vi "MoD Main-Optimize - HPLC BH-Amination - ReOpt.vi"() -> ()   [LabVIEW 2015]
uses:
  <vilib>/silver_ctls/ArrayMatrixCluster/Real Matrix NI_Silver.ctl
  <vilib>/ni845x/ni845x.llb/ni845xControl.ctl
  <vilib>/MakerHub/LINX/Public/Peripherals/Analog/Analog Read 1 Chan.vi
  <vilib>/MakerHub/LINX/Public/Peripherals/Analog/Analog Read N Chans.vi
  <vilib>/MakerHub/LINX/Public/Peripherals/Digital/Digital Write 1 Chan.vi
  <vilib>/MakerHub/LINX/Private/Local IO/LinxAnalogRead.vi
  <vilib>/MakerHub/LINX/Public/Utilities/Check Channel.vi
  <vilib>/MakerHub/LINX/Public/Peripherals/Digital/Digital Write N Chans.vi
  <vilib>/MakerHub/LINX/Private/Local IO/LinxDigitalWrite.vi
  <vilib>/addons/control/pid/pid.llb/PID Control Input Filter (DBL).vi
  <vilib>/MakerHub/LINX/Private/Utilties/Generate Error.vi
  <vilib>/addons/control/pid/autopid.llb/PID Online Autotuning (Relay Feedback).vi
  <vilib>/Analysis/Matrix/Numeric/Conversions/Array To Matrix - RA2.vi
  <vilib>/ni845x/ni845x.llb/NI-845x Close Device Reference.vi
  <vilib>/addons/control/pid/NI_PID_autopid.lvlib
  <vilib>/addons/control/pid/NI_PID_pid.lvlib
  <vilib>/Analysis/Matrix/NI_Matrix.lvlib
  <vilib>/MakerHub/LINX/LMH-LINX.lvlib
  <instrlib>/Harvard Apparatus PHD Ultra Series/Harvard Apparatus PHD Ultra Series.lvlib
panel:
  out "running?":bool=TRUE
  out "new_reactor_volume":bool[](array[boolean])
  out "new_reactor_length":bool[](array[boolean])
  out "Phase_Sensor_voltage":dbl
  out "P_tot":dbl
  out "pause for ms":bool=TRUE
  out "stop_xl_write":bool=TRUE
  out "Num_exp_till_pause":i32
  out "Syringe_pump?":bool=TRUE
  out "System Error":bool=TRUE
  out "error out":errorcluster
  out "Pump setpoint(ul/min) 6":dbl format="%#_13g"
  out "Pump setpoint(ul/min) 5":dbl format="%#_13g"
  out "Pump setpoint(ul/min) 4":dbl format="%#_13g"
  out "Pump setpoint(ul/min) 3":dbl format="%#_13g"
  out "Pump setpoint(ul/min) 2":dbl format="%#_13g"
  out "Pump setpoint(ul/min) 1":dbl format="%#_13g"
  out "Volume (ul) 5":dbl format="%#_13g"
  out "Volume (ul) 4":dbl format="%#_13g"
  out "Volume (ul) 3":dbl format="%#_13g"
  out "Volume (ul) 2":dbl format="%#_13g"
  out "Volume (ul) 1":dbl format="%#_13g"
  in  "tau 5":dbl format="%#_13g"
  out "tau 4":dbl format="%#_13g"
  out "tau 3":dbl format="%#_13g"
  out "tau 2":dbl format="%#_13g"
  out "tau 1":dbl format="%#_13g"
  out "Reactor Length":dbl format="%#_13g"
  out "Flowrate Sensor 2":dbl format="%#_13g"
  out "Flowrate Sensor 1":dbl format="%#_13g"
  out "Pressure 2":dbl format="%#_13g"
  out "Pressure 1":dbl format="%#_13g"
  out "Temperature Control 5":bool=TRUE
  out "Temperature Control 4":bool=TRUE
  out "Temperature Control 3":bool=TRUE
  out "Temperature Control 2":bool=TRUE
  out "Temperature Control 1":bool=TRUE
  out "Temperature SP 5":dbl format="%#_g'C"
  out "Temperature SP 4":dbl format="%#_g'C"
  out "Temperature SP 3":dbl format="%#_g'C"
  out "Temperature SP 2":dbl format="%#_g'C"
  out "Temperature SP 1":dbl format="%#_g'C"
  in  "Bay Temperature 5":dbl
  in  "SSR Duration 5":dbl
  in  "SSR Duration 4":dbl
  in  "SSR Duration 3":dbl
  in  "SSR Duration 2":dbl
  in  "SSR Duration 1":dbl
  in  "Total Product Amount":dbl=1.0 format="%#_gml"
  out "Setup Error":bool=TRUE
  out "Error Message":string
  out "ID CTR":i32
  in  "Tab Control":T1(tab)
  out "Reagent pic 5":picture
  in  "reagent name 5":string="toluene"
  out "Reagent Pic 4":picture
  in  "reagent name 4":string="sodium hydroxide"
  out "Reagent Pic 3":picture
  in  "reagent  name 3":string="1470372-59-8"
  in  "Product name":string="101-70-2"
  in  "reagent name 1":string="4-bromoanisole"
  out "Reagent Pic 1":picture
  in  "Vr5":dbl format="%#_guL"
  in  "Vr4":dbl format="%#_guL"
  in  "Vr3":dbl format="%#_guL"
  in  "Vr2":dbl format="%#_guL"
  in  "Vr1":dbl format="%#_guL"
  in  "System decide help Button":bool
  in  "Reaction Scheme Confirm":bool
  in  "Synthesis Route Array":string[][](array[string])=[["4-bromoanisole + naphtalene (0.5M)", "1", "PhB(OH)2", "", "", ""], ["p-anisidine", "1", "-", "-", "-", "-"], ["Brettphos PdG3", "0.0025", "-", "-", "-", "-"], ["NaOH", "1", "-", "-", "-", "-"], ["Toluene", "8", "-", "-", "-", "-"], ["Water", "8", "-", "-", "-", "-"]]
  in  "System decide help Button 2":bool
  out "Setup Confirm":bool=TRUE
  in  "BAY 1":u16(ring) items=["               Bypass", "         Heated Reactor", "    Small Heated Reator", "         Cooled Reactor", "      Packed Bed Reactor", "          Photo Reactor", "             Separator"]
  in  "BAY 5":u16(ring)=6 items=["               Bypass", "         Heated Reactor", "    Small Heated Reactor", "         Cooled Reactor", "     Packed Bed Reactor", "         Photo Reactor", "             Separator"]
  in  "BAY 4":u16(ring) items=["                Bypass", "         Heated Reactor", "    Small Heated Reactor", "         Cooled Reactor", "     Packed Bed Reactor", "         Photo Reactor", "             Separator"]
  in  "BAY 3":u16(ring)=1 items=["               Bypass", "         Heated Reactor", "    Small Heated Reactor", "         Cooled Reactor", "     Packed Bed Reactor", "          Photo Reactor", "             Separator"]
  in  "BAY 2":u16(ring) items=["               Bypass", "         Heated Reactor", "    Small Heated Reactor", "         Cooled Reactor", "      Packed Bed Reactor", "          Photo Reactor", "             Separator"]
  out "Reagent Pic 2":picture
  out "Product Pic":picture
  in  "reagent name 2":string="p-anisidine"
  in  "reagent name 6":string="water"
  out "Reagent Pic 6":picture
  in  "System Parameters Help Button":bool
  out "Setup Confirm 2":bool
  in  "System Parameters Confirm Button":bool
  in  "Bay Parameters":T2={"Bay 1 "={"Pump 1 Flowrate"=0.0, "optimize_temp"=FALSE, "optimize_tau"=TRUE, "Run at set flowrate"=FALSE, "Pump 2 Flowrate"=0.0, "Temperature Params"=[40.0, 100.0, 100.0], "pump params 1"=[16.3, 65.9, 325.0], "pump params 2"=[16.3, 65.9, 325.0], "Temperature"=0.0, "Run at set temperature"=FALSE}, "Bay 2 "={"Pump 3 Flowrate"=0.5, "optimize_temp"=FALSE, "optimize_tau"=FALSE, "Run at set flowrate"=TRUE, "Temperature Params"=[40.0, 100.0, 100.0], "Resisdence time params"=[0.1, 2.0, 650.0], "pump_at_ratio"=FALSE, "pump_num_ratio"=4.0, "Temperature"=0.0, "Run at set temperature"=FALSE}, "Bay 3 "={"Pump 4 Flowrate"=100.0, "optimize_temp"=FALSE, "optimize_tau"=TRUE, "Run at set flowrate"=FALSE, "Temperature Params"=[40.0, 100.0, 100.0], "Resisdence time params"=[16.3, 65.9, 0.0], "pump_at_ratio"=FALSE, "pump_num_ratio"=0.0, "Temperature "=100.0, "Run at set temperature"=TRUE}, "Bay 4 "={"Pump 5 Flowrate"=40.0, "Run at set flowrate"=FALSE, "optimize_temp"=FALSE, "optimize_tau"=FALSE, "Resisdence time params"=[40.6, 406.0, 225.0], "Temperature Params"=[40.0, 100.0, 80.0], "pump_at_ratio"=TRUE, "pump_num_ratio"=1.0, "Temperature"=0.0, "Run at set temperature"=FALSE}, "Bay 5 "={"Pump 6 Flowrate"=0.0, "Run at set flowrate"=FALSE, "optimize_temp"=FALSE, "optimize_tau"=FALSE, "Resisdence time params"=[7.62, 114.27, 0.0], "Temperature Params"=[0.0, 0.0, 0.0], "pump_at_ratio"=TRUE, "pump_num_ratio"=0.5, "Temperature"=0.0, "Run at set temperature"=FALSE}, "Excel File Name"="C:\\Users\\HPLC\\Dropbox (MIT)\\MoD Files\\Data\\BHamination07252017", "hplc File Name"="C:\\Chem32\\1\\Data\\MOD", "Matlab File"="C:\\Users\\HPLC\\Dropbox (MIT)\\MoD Files\\Data\\BHamination07252017", "Syringe for Pump 2?"=TRUE, "Num_conditons_per_wait"=2.0, "Continue from previous optimization?"=FALSE, "Total Number of Experiments 2"=15.0, "Hplc Wait time(min)"=5.0, "increas_decrease_hplc_peak"=TRUE, "Internal Standard?"=TRUE, "ISTD start"=3.7, "ISTD end"=5.0, "hplc_start"=3.0, "hplc_end"=4.0, "throughput_yield"=TRUE} {"Hplc Wait time(min)" format="%#_13g"; "Bay 5"."Temperature Params" format="%#_g'C"; "Bay 4"."Temperature Params" format="%#_g'C"; "Bay 3"."Temperature Params" format="%#_g'C"; "Bay 2"."Temperature Params" format="%#_g'C"; "Bay 1"."Temperature Params" format="%#_g'C"}
  out "System Confirm Not Clicked":string
  out "best_exp_num":dbl=1.0
  out "temperature_best":dbl[](array[numeric])
  out "Flowrates(ul/min)_best":dbl[](array[numeric])
  out "System Status":u16(ring)=2 caption="Sy" items=["System  Error", "System Running", "System Standby"]
  out "Current Experiment":dbl=1.0
  out "Total Number of Experiments":dbl=33.0
  out "Phase Sensor Chart":T3(graph)
  out "HPLC Analysis":bool
  out "Equlibrating Temperature":bool
  out "Flushing System":bool
  out "Calculate condition":bool
  out "Temperature 5":dbl format="%#_g'C"
  out "Temperature 4":dbl format="%#_g'C"
  out "Temperature 3":dbl format="%#_g'C"
  out "Temperature 2":dbl format="%#_g'C"
  out "Temperature 1":dbl format="%#_g'C"
  out "Flowrate Chart":T4(graph)
  out "Teperature Chart":T3(graph)
  out "Pump Setpoints Chart":T3(graph)
  out "Pressure Chart":T3(graph)
  out "Optimization_loop_index":i32
  out "curr_wait_time":dbl
  out "total_flush_time":dbl
  out "Temp SS? 5":bool=TRUE
  out "Temp SS? 4":bool=TRUE
  out "Temp SS? 3":bool=TRUE
  out "Temp SS? 2":bool=TRUE
  out "Temp SS? 1":bool=TRUE
  out "System Flushed?":bool
  out "stop_button clicked":bool
  out "experiment history":T5
  in  "Number of System Flushes per condtion":dbl=2.5
  in  "calculate volume 3":bool
  in  "calculate volume 2":bool=TRUE
  in  "calculate volume 1":bool=TRUE
  in  "calculate volume 4":bool
  in  "calculate volume 5":bool
  in  "Extra system dead volume":dbl format="%#_gul"
  in  "new reactor length? 1":bool
  in  "tube_length(in)":dbl[](array[numeric])=[188.0, 188.0, 10.0, 10.0, 10.0]
  out "Pause Before Analysis":bool
  out "Chiller COMM Port":bool
  out "Arduino COMM Port 2":bool
  out "Temperature Sensor COMM Port":bool
  out "Flow Rate":bool
  out "Pressure":bool
  out "Pump COMM Port":bool
  in  "COMM Port :: Milligat Pumps":refnum<visa-resource-name>="COM10"
  in  "Arduino COMM Port":refnum<visa-resource-name>="COM3"
  in  "Sample Valve COMM::Port":refnum<visa-resource-name>="COM6"
  in  "COMM Port:: Harvard Syringe Pump":refnum<visa-resource-name>="COM5"
  in  "tube_id(in)":enum16{".01", ".02", ".03", ".04"}[](array[ring])=[enum.".03", enum.".03", enum.".03", enum.".03", enum.".03"]
  out "Total System Resisdence Time(min)":dbl
  in  "Debug_run_button":bool
  in  "new reactor length? 2":bool
  in  "new reactor length? 3":bool
  in  "new reactor length? 4":bool
  in  "new reactor length? 5":bool
  in  "IR Sensor Device":T6="USB0::0x3923::0x7514::01B3FF21::RAW"
  out "Stop":bool=TRUE
  in  "Run_Stop_cluster":T7
  # "Molecules on Demand"
  # "Synthetic Route"
  # "5"
  # "6"
  # "4"
  # "Product"
  # "1"
  # "2"
  # "3"
  # "Reagent List"
  # "Concentration(M)"
  # "Molecule"
  # "1"
  # "1"
  # "2"
  # "2"
  # "3"
  # "3"
  # "4"
  # "4"
  # "5"
  # "6"
  # "5"
  # "6"
  # "Product"
  # "Reactor Volume:"
  # "Optimization Parameters"
  # "Pause after"
  # "Experiments"
  # "Optimize for"
  # "to"
  # "of HPLC Peak from"
  # "from"
  # "to"
  # "min"
  # "min"
  # "HPLC runtime"
  # "# Iterations"
  # "Reporting"
  # "Excel Output File Name"
  # "HPLC File Path"
  # "MATLAB File Path"
  # "Temperature"
  # "Flowrate(ul/min)"
  # "Lower Bound"
  # "Upper Bound"
  # "Optimize?"
  # "-or-"
  # "Run at"
  # "times incoming flow"
  # "Setpoint"
  # "Temperature"
  # "Flowrate(ul/min)"
  # "Lower Bound"
  # "Upper Bound"
  # "Optimize?"
  # "-or-"
  # "Run at"
  # "times incoming flow"
  # "Setpoint"
  # "Temperature"
  # "Flowrate(ul/min)"
  # "Lower Bound"
  # "Upper Bound"
  # "Optimize?"
  # "-or-"
  # "Run at"
  # "times incoming flow"
  # "Setpoint"
  # "Temperature"
  # "Flowrate 3 (ul/min)"
  # "Lower Bound"
  # "Upper Bound"
  # "Optimize?"
  # "-or-"
  # "Run at"
  # "times incoming flow"
  # "Setpoint"
  # "Temperature"
  # "Flowrate 1(ul/min)"
  # "Flowrate 2(ul/min)"
  # "Lower Bound"
  # "Upper Bound"
  # "Optimize?"
  # "Setpoint"
  # "Pressure (psi)"
  # "System Status"
  # "Temperature('C)"
  # "BAY"
  # "1"
  # "2"
  # "3"
  # "4"
  # "5"
  # "Pump Flowrate Setpoint(ul/min)"
  # "Flowrate (ul/min)"
  # "Phase Sensor"
  # "Current Experiment"
  # "Temperature('C)"
  # "Flowrate(ul/min)"
  # "Exp"
  # "Current Best Condition"
  # "Time to reach steady state:"
  # "Current Wait Time:"
  # "Experimental Steps"
  # "Calculated New Conditions"
  # "Steady State"
  # "Analyzed HPLC"
  # "Equilibrated Temperature"
  # "Tube Length (cm)"
  # "Bay"
  # "Tube ID (in)"
  # "Calculate Volume"
  # "Use new tube length"
  # "1."
  # "2."
  # "3."
  # "4."
  # "5."
  # "Reactor Lengths\n*Heated Reactor - 188cm * Small Reactor - 99cm * Bypass - 10cm * Separator - *"
  # "All Experimental Data"
  # "P1"
  # "P2"
  # "P3"
  # "P4"
  # "P5"
  # "P6"
  # "T1"
  # "T2"
  # "T3"
  # "T4"
  # "T5"
  # "Obj_fun"
  # "HPLC_Data"
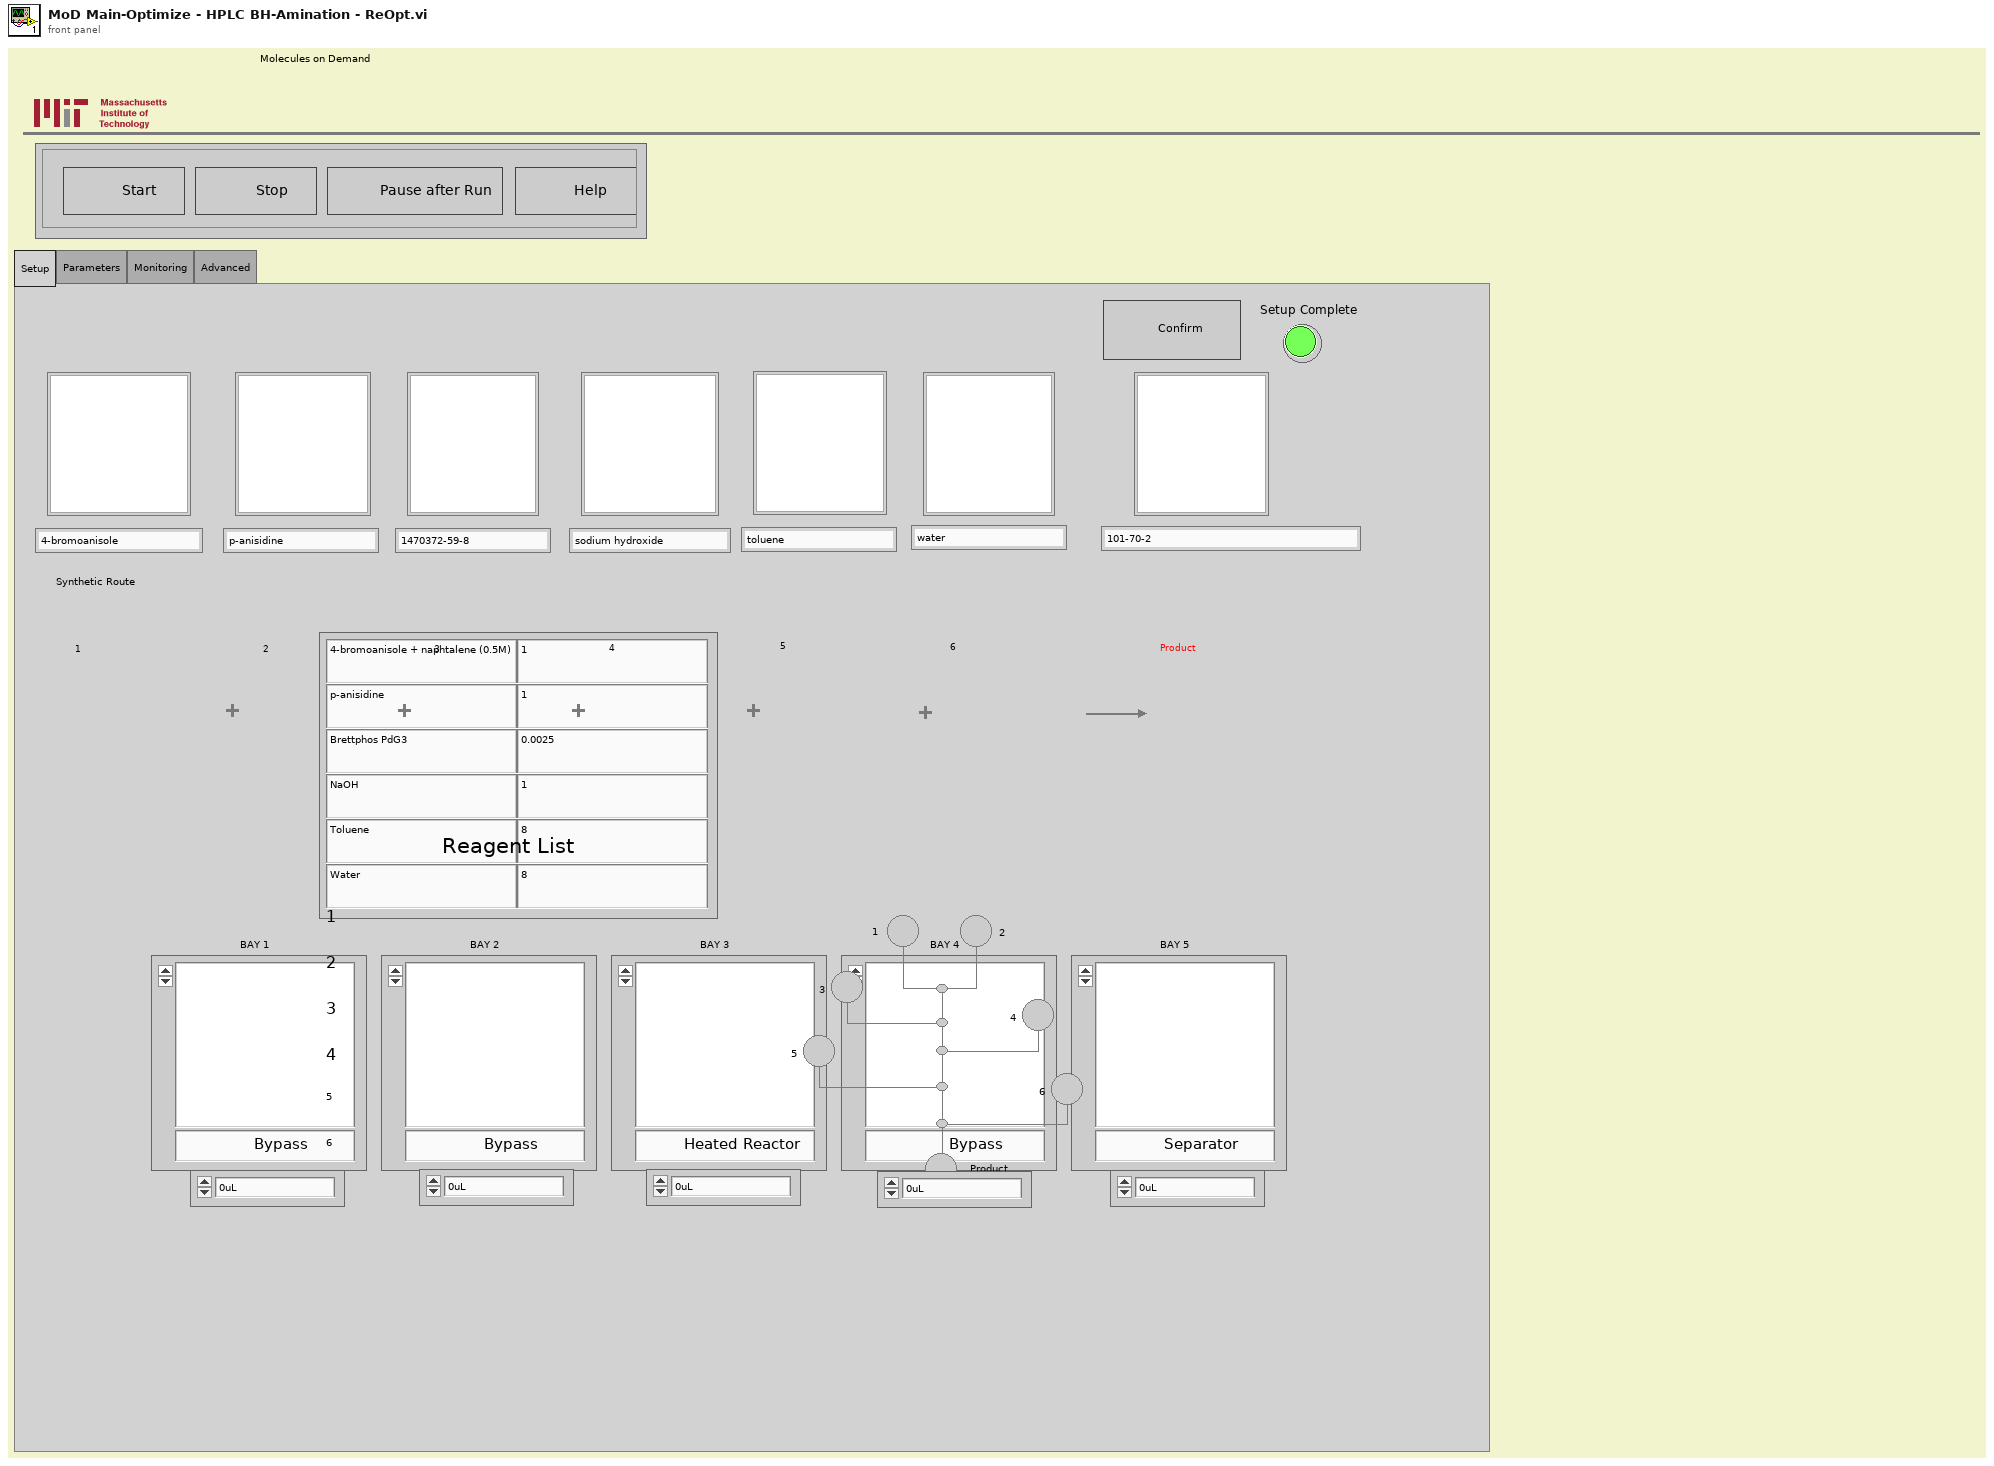
[diagram p1: front panel]
types:
  T1 = enum32{"Setup", "Parameters", "Monitoring", "Advanced"}
  T2 = cluster{"Bay 1 ":cluster{"Pump 1 Flowrate":dbl, "optimize_temp":bool, "optimize_tau":bool, "Run at set flowrate":bool, "Pump 2 Flowrate":dbl, "Temperature Params":dbl[], "pump params 1":dbl[], "pump params 2":dbl[], "Temperature":dbl, "Run at set temperature":bool}, "Bay 2 ":cluster{"Pump 3 Flowrate":dbl, "optimize_temp":bool, "optimize_tau":bool, "Run at set flowrate":bool, "Temperature Params":dbl[], "Resisdence time params":dbl[], "pump_at_ratio":bool, "pump_num_ratio":dbl, "Temperature":dbl, "Run at set temperature":bool}, "Bay 3 ":cluster{"Pump 4 Flowrate":dbl, "optimize_temp":bool, "optimize_tau":bool, "Run at set flowrate":bool, "Temperature Params":dbl[], "Resisdence time params":dbl[], "pump_at_ratio":bool, "pump_num_ratio":dbl, "Temperature ":dbl, "Run at set temperature":bool}, "Bay 4 ":cluster{"Pump 5 Flowrate":dbl, "Run at set flowrate":bool, "optimize_temp":bool, "optimize_tau":bool, "Resisdence time params":dbl[], "Temperature Params":dbl[], "pump_at_ratio":bool, "pump_num_ratio":dbl, "Temperature":dbl, "Run at set temperature":bool}, "Bay 5 ":cluster{"Pump 6 Flowrate":dbl, "Run at set flowrate":bool, "optimize_temp":bool, "optimize_tau":bool, "Resisdence time params":dbl[], "Temperature Params":dbl[], "pump_at_ratio":bool, "pump_num_ratio":dbl, "Temperature":dbl, "Run at set temperature":bool}, "Excel File Name":string, "hplc File Name":string, "Matlab File":string, "Syringe for Pump 2?":bool, "Num_conditons_per_wait":dbl, "Continue from previous optimization?":bool, "Total Number of Experiments 2":dbl, "Hplc Wait time(min)":dbl, "increas_decrease_hplc_peak":bool, "Internal Standard?":bool, "ISTD start":dbl, "ISTD end":dbl, "hplc_start":dbl, "hplc_end":dbl, "throughput_yield":bool}
  T3 = cluster{"[0]":dbl, "[1]":dbl, "[2]":dbl, "[3]":dbl, "[4]":dbl, "[5]":dbl, "[6]":dbl, "[7]":dbl, "[8]":dbl}
  T4 = cluster{"[0]":i32, "[1]":i32, "[2]":i32, "[3]":i32, "[4]":i32, "[5]":i32, "[6]":i32, "[7]":i32, "[8]":i32}
  T5 = typedef "Real Matrix NI_Silver.ctl" = dbl[][]
  T6 = typedef "ni845xControl.ctl" = refnum<k21>
  T7 = cluster{"Stop":bool, "Run":bool, "Stop Run Button":bool, "Help Button":bool}
  T8 = cluster{"Proportional gain Kc":dbl, "Integral time Ti (sec)":dbl, "Derivative time Ti (sec)":dbl}
  T9 = cluster{"type of controller":enum16{"P", "PI", "PID"}, "relay cycles":i32, "relay amplitude":dbl, "control specifications":enum16{"Fast", "Normal", "Slow"}, "PV noise level":dbl}
  T10 = typedef "LMH-LINX.lvlib/LINX Ref.ctl" = cluster{"IO":T11, "Interface":T12, "LINX Device Config":T13}
  T11 = typedef "LMH-LINX.lvlib/Platform.ctl" = enum16{"Remote", "Local"}
  T12 = typedef "LMH-LINX.lvlib/Interface.ctl" = enum16{"Serial", "TCP"}
  T13 = typedef "LMH-LINX.lvlib/Device.lvlib/LINX Device Config.ctl" = cluster{"Interface":T12, "COM Port":refnum<visa-resource-name>, "TCP Configuration":T14, "Device Family":u8, "Device ID":u8, "Device Name":string, "TCP Ref":refnum<k5>, "Channels":T15}
  T14 = typedef "LMH-LINX.lvlib/Device.lvlib/TCP Config.ctl" = cluster{"IP Address":string, "Port":u16}
  T15 = typedef "LMH-LINX.lvlib/Channels.ctl" = cluster{"DI":u8[], "DO":u8[], "AI":u8[], "AO":u8[], "PWM":u8[], "QE":u8[], "UART":u8[], "I2C 2":u8[], "SPI":u8[], "CAN":u8[], "Servo":u8[], "AI Ref (V)":dbl, "AI Resolution (Bits)":u8, "AO Ref (V)":dbl, "AO Resolution (Bits)":u8}
  T16 = typedef "imagedata.ctl" = cluster{"image type":i32, "image depth":i32, "image":u8[], "mask":u8[], "colors":u32[], "Rectangle":cluster{"left":i16, "top":i16, "right":i16, "bottom":i16}}
  T17 = cluster{"proportional gain (Kc)":dbl, "integral time (Ti, min)":dbl, "derivative time (Td, min)":dbl}
  T18 = typedef "NI_Matrix.lvlib/RealMatrix.ctl" = dbl[][]
  T19 = enum16{"Left Button", "Center Button", "Right Button", "Window Close"}
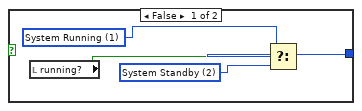
[diagram p3: hidden frame]
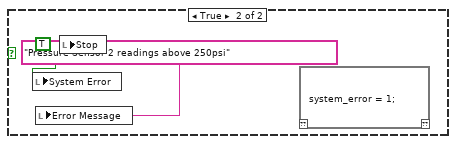
[diagram p4: hidden frame]
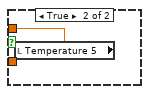
[diagram p6: hidden frame]
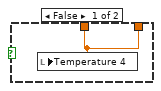
[diagram p7: hidden frame]
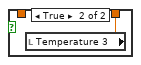
[diagram p8: hidden frame]
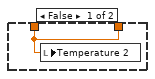
[diagram p9: hidden frame]
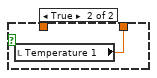
[diagram p10: hidden frame]
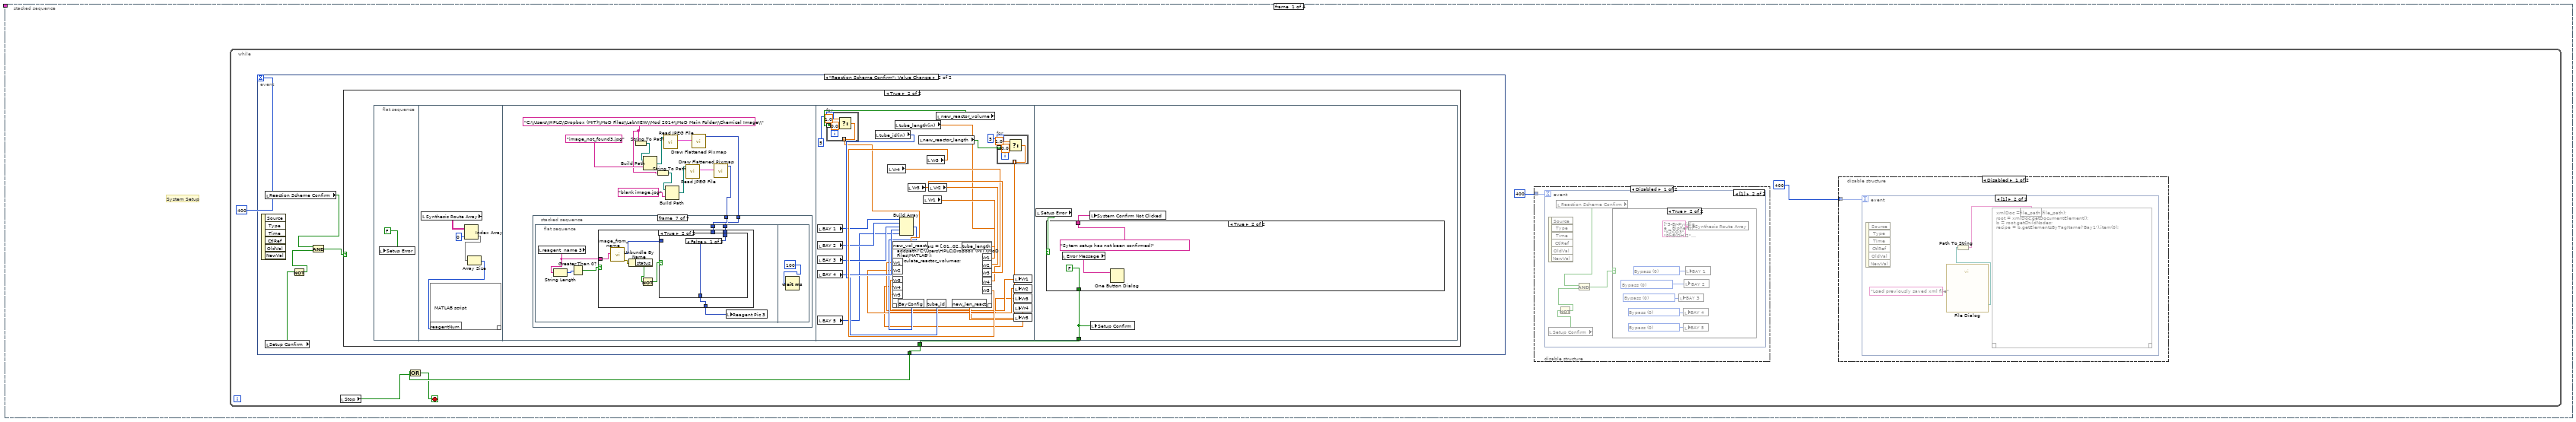
[diagram p11: hidden frame]
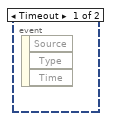
[diagram p12: hidden frame]
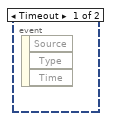
[diagram p14: hidden frame]
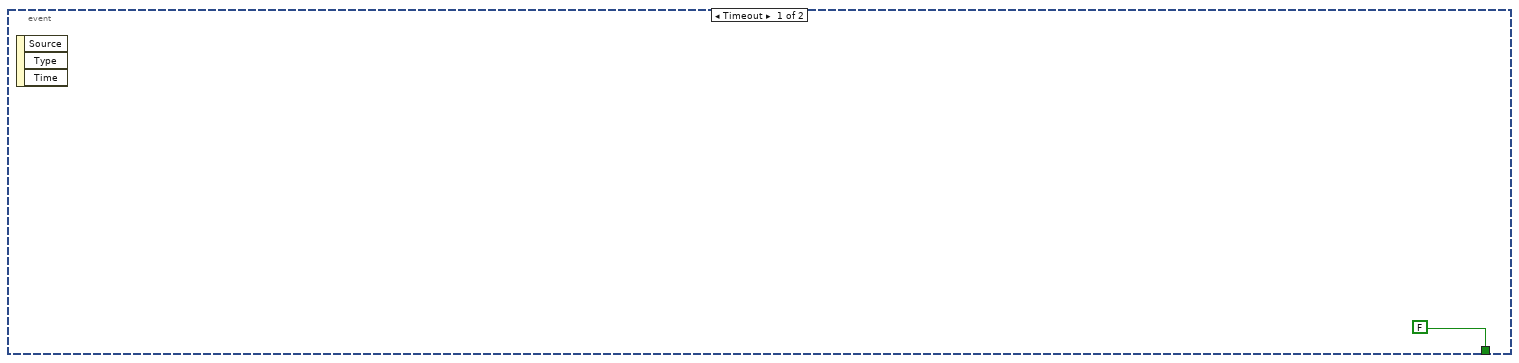
[diagram p17: hidden frame]
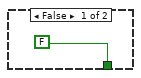
[diagram p18: hidden frame]
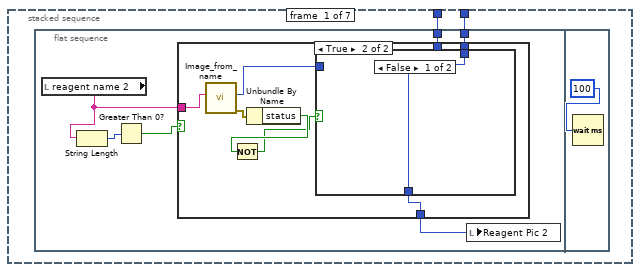
[diagram p19: hidden frame]
diagram:
  # "Assume User always uses the first bay first"
  n1 = flat-sequence {
    tunnel: ["COMM Port :: Milligat Pumps"] -> w9
    tunnel: ["Arduino COMM Port"] -> w8
    tunnel: [w11] -> w5
    tunnel: ["Bay Parameters"] -> w4
    tunnel: [w60] -> w10
    tunnel: w9 -> [w60]
    tunnel: w8 -> [w48]
    tunnel: [w54] -> w7
    tunnel: [w52] -> w6
    tunnel: w5 -> [w52]
    tunnel: w4 -> [w50]
    tunnel: [w47] -> w3
    tunnel: w10 -> [w66]
    tunnel: w7 -> [w65]
    tunnel: w6 -> [w63]
    tunnel: w3 -> [w61]
    tunnel: [w61] -> w1
    tunnel: [w1358] -> w2
    tunnel: w1 -> [w1358]
    tunnel: w2 -> [w1359]
    frame #0 {
      w36 = FALSE ("Equlibrating Temperature")
      n2 = script code="TempArr1=[23 23 23 23 23 23 23 23 23 23]';\nTempArr2=[23 23 23 23 23 23 23 23 23 23]';\nTempArr3=[23 23 23 23 23 23 23 23 23 23]';\nTempArr4=[23 23 23 23 23 23 23 23 23 23]';\nTempArr5=[23 23 23 23 23 23 23 23 23 23]';\ntemp_error1 =0;\ntemp_error2 =0;\ntemp_error3 =0;\ntemp_error4 =0;\ntemp_error5 =0;\ntemp_check1 = 0;\ntemp_check2 = 0;\ntemp_check3 = 0;\ntemp_check4 = 0;\ntemp_check5 = 0;\nT1=23;\nT2=23;\nT3=23;\nT4=23;\nT5=23;"() -> ()  [unwired: 1 in, 1 out]
      n3 = Build Array("calculate volume 1", "calculate volume 2", "calculate volume 3", "calculate volume 4", "calculate volume 5") -> (→"new_reactor_volume":bool[])
      n4 = Build Array("new reactor length? 1", "new reactor length? 2", "new reactor length? 3", "new reactor length? 4", "new reactor length? 5") -> (→"new_reactor_length":bool[])
      n5 = call <vilib>:"Initialize.vi"("VISA resource name"="COMM Port:: Harvard Syringe Pump") -> ("VISA resource name out"=w11:refnum<visa-resource-name>)  [unwired: 9 in, 1 out]
      "Stop" <- FALSE ("Stop")
      "ID CTR" <- 0
      "Setup Confirm" <- FALSE ("Setup Confirm")
      "Error Message" <- "System shutdown sucessfully. No errors to report." ("Error Message")
      "Setup Error" <- FALSE ("Setup Error")
      "Reactor Length" <- 10.5
      "System Error" <- FALSE ("System Error")
      "Num_exp_till_pause" <- 0 ("Num_exp_till_pause")
      "Equlibrating Temperature" <- w36
      "Calculate condition" <- w36
      "Flushing System" <- w36
      "HPLC Analysis" <- w36
      "stop_xl_write" <- FALSE ("stop_xl_write")
      "Pump setpoint(ul/min) 1" <- 0.0 ("Pump setpoint(ul/min) 1")
      "Pump setpoint(ul/min) 2" <- 0.0 ("Pump setpoint(ul/min) 2")
      "Pump setpoint(ul/min) 4" <- 0.0 ("Pump setpoint(ul/min) 4")
      "Pump setpoint(ul/min) 6" <- 0.0 ("Pump setpoint(ul/min) 6")
      "Pump setpoint(ul/min) 3" <- 0.0 ("Pump setpoint(ul/min) 3")
      "Pump setpoint(ul/min) 5" <- 0.0 ("Pump setpoint(ul/min) 5")
      "pause for ms" <- FALSE ("pause for ms")
      "Setup Confirm 2" <- FALSE ("Setup Confirm 2")
      "running?" <- FALSE ("running?")
    }
    frame #1 {
      w49 = FALSE
      w59 = 23
      (unwired) path "C:/Users/User1/Documents/Lab/MoD/Images"
      n6 = disable-structure shown="Disabled" {
        frame Disabled {
          n7 = local read "BAY 2"() -> ()  [unwired: 1 out]
          n8 = local read "BAY 3"() -> ()  [unwired: 1 out]
          n9 = local read "BAY 4"() -> ()  [unwired: 1 out]
          n10 = local read "BAY 5"() -> ()  [unwired: 1 out]
          n11 = local read "BAY 1"() -> ()  [unwired: 1 out]
        }
        frame Enabled {
        }
      }
      n12 = local write "Debug_run_button"(TRUE) -> ()
      n13 = call <vilib>:"Initialize.vi"("Serial Port"=w48) -> ("LINX Resource"=w47:T10)  [unwired: 8 in, 2 out]
      n14 = local write "System Parameters Confirm Button"(w49) -> ()
      n15 = local write "Setup Confirm 2"(w49) -> ()
      n16 = Unbundle By Name(w50) -> ("Syringe for Pump 2?"=→"Syringe_pump?":bool)
      n17 = local write "Temperature 1"(w59) -> ()
      n18 = local write "Temperature 2"(w59) -> ()
      n19 = local write "Temperature 3"(w59) -> ()
      n20 = local write "Temperature 4"(w59) -> ()
      n21 = local write "Temperature 5"(w59) -> ()
      n22 = local write "Temperature SP 1"(w59) -> ()
      n23 = local write "Temperature SP 2"(w59) -> ()
      n24 = local write "Temperature SP 3"(w59) -> ()
      n25 = local write "Temperature SP 4"(w59) -> ()
      n26 = local write "Temperature SP 5"(w59) -> ()
      n27 = Current VI's Path() -> (path=w58:path)
      n28 = Strip Path(path=w58) -> (stripped path=w56:path)  [unwired: 1 out]
      n29 = Strip Path(path=w56) -> (stripped path=w55:path)  [unwired: 1 out]
      n30 = Build Path(base path=w55, name or relative path="MATLAB") -> (appended path=w54:path)
    }
    frame #2 {
      # "Main Help Dialog Popup"
      n31 = while {
        stop <- w1352 stop-if-true
        n32 = event shown="[6] \"Run_Stop_cluster.Run\": Value Change" {
          selector: _ -> [_ _ _ _ _ _ _]
          dyn-events: _ -> [_ _ _ _ _ _ _]
          timeout: 100 -> [_ _ _ _ _ _ _]
          event Timeout {
            n33 = event-data() -> ()  [unwired: 1 in, 3 out]
          }
          event "Run_Stop_cluster.Help Button": Value Change {
            n34 = local read "Run_Stop_cluster"() -> (w1355:T7)
            n35 = event-data() -> ()  [unwired: 1 in, 4 out]
            n36 = Unbundle By Name(w1355) -> ("Help Button"=w1354:bool)
            n37 = case shown="True" w1354 {
              frame False {
              }
              frame True {
                n38 = call "help.vi"() -> ()  [unwired: 11 in]
              }
            }
          }
          event "System decide help Button": Value Change {
            n39 = event-data() -> ()  [unwired: 1 in, 5 out]
            n40 = call "help_synthesis_man-auto_instructions.vi"() -> ()  [unwired: 12 in]
          }
          event "System Parameters Help Button": Value Change {
            n41 = event-data() -> ()  [unwired: 1 in, 5 out]
            n42 = call "help_parameters_setup.vi"() -> ()  [unwired: 12 in]
          }
          event "System decide help Button 2": Value Change {
            n43 = event-data() -> ()  [unwired: 1 in, 5 out]
            n44 = call "help_synthesis_route_instructions.vi"() -> ()  [unwired: 12 in]
          }
          event "Run_Stop_cluster.Stop": Value Change {
            n45 = event-data() -> ()  [unwired: 1 in, 5 out]
            n46 = local write "Stop"(TRUE) -> ()
          }
          event "Run_Stop_cluster.Run": Value Change {
            n47 = event-data() -> ()  [unwired: 1 in, 5 out]
            n48 = local write "running?"(TRUE) -> ()
          }
        }
        n49 = local read "Stop"() -> (w1352:bool)
      }
      n50 = stacked-sequence {
        tunnel: w66 -> [_ _ _ _]
        tunnel: w65 -> [_ w425 _ _]
        tunnel: w63 -> [_ _ _ w592]
        tunnel: w61 -> [_ _ _ w590]
        frame #0 {
          # "System Setup"
          n51 = while {
            stop <- w200 stop-if-true
            n52 = event shown="[1] \"Reaction Scheme Confirm\": Value Change" {
              selector: _ -> [_ _]
              dyn-events: _ -> [_ _]
              timeout: 400 -> [_ _]
              tunnel: [FALSE w220] -> w202
              event Timeout {
                n53 = event-data() -> ()  [unwired: 1 in, 3 out]
              }
              event "Reaction Scheme Confirm": Value Change {
                n54 = event-data() -> ()  [unwired: 1 in, 6 out]
                n55 = local read "Reaction Scheme Confirm"() -> (w224:bool)
                n56 = local read "Setup Confirm"() -> (w222:bool)
                n57 = Not(x=w222) -> (.not. x?=w221:bool)
                n58 = And(x=w224, y=w221) -> (x .and. y?=w223:bool)
                n59 = case shown="True" w223 {
                  tunnel: [FALSE w226] -> w220
                  frame False {
                  }
                  frame True {
                    n60 = flat-sequence {
                      tunnel: [w415] -> w226
                      frame #0 {
                        n61 = local write "Setup Error"(FALSE) -> ()
                      }
                      frame #1 {
                        n62 = local read "Synthesis Route Array"() -> (w230:string[][])
                        n63 = Index Array(array=w230, index (col)=0 ("disabled index (col)")) -> (element=w228:string[])  [unwired: 1 in]
                        n64 = Array Size(array=w228) -> (size(s)=w231:i32)
                        n65 = script code="MATLAB script"("reagentNum"=w231) -> ()  [unwired: 1 in, 1 out]
                      }
                      frame #2 {
                        w234 = "C:\\Users\\HPLC\\Dropbox (MIT)\\MoD Files\\LabVIEW\\Mod 2014\\MoD Main Folder\\Chemical Image\\" ("string")
                        n66 = String To Path(string=w234) -> (path=w240:path)
                        n67 = Build Path(base path=w240, name or relative path="image_not_found3.jpg") -> (appended path=w239:path)
                        n68 = String To Path(string=w234) -> (path=w237:path)
                        n69 = call <vilib>:"Read JPEG File.vi"("path to JPEG file"=w239) -> ("image data"=w242:T16)  [unwired: 1 in, 9 out]
                        n70 = Build Path(base path=w237, name or relative path="blank image.jpg") -> (appended path=w235:path)
                        n71 = call <vilib>:"Read JPEG File.vi"("path to JPEG file"=w235) -> ("image data"=w238:T16)  [unwired: 1 in, 9 out]
                        n72 = call <vilib>:"Draw Flattened Pixmap.vi"("image data"=w242) -> ("new picture"=w233:picture)  [unwired: 3 in, 5 out]
                        n73 = call <vilib>:"Draw Flattened Pixmap.vi"("image data"=w238) -> ("new picture"=w232:picture)  [unwired: 3 in, 5 out]
                        n74 = stacked-sequence {
                          tunnel: w233 -> [w244 w264 w284 w304 w324 w343 w363]
                          tunnel: w232 -> [w243 w263 w283 w303 w323 w344 w364]
                          frame #0 {
                            n75 = flat-sequence {
                              tunnel: w244 -> [w250]
                              tunnel: w243 -> [w248]
                              frame #0 {
                                n76 = local read "reagent name 2"() -> (w246:string)
                                n77 = String Length(string=w246) -> (length=w249:i32)
                                n78 = Greater Than 0?(x=w249) -> (x > 0?=w247:bool)
                                n79 = case shown="True" w247 {
                                tunnel: w250 -> [_ w256]
                                tunnel: w248 -> [w251 _]
                                tunnel: [w251 w255] -> w245
                                tunnel: w246 -> [_ w254]
                                frame False {
                                }
                                frame True {
                                n80 = call "Image_from_name.vi"("Chemical Name"=w254) -> ("error out"=w257:errorcluster, "Downloaded Picture"=w258:picture)  [unwired: 8 in, 1 out]
                                n81 = Unbundle By Name(w257) -> ("status"=w253:bool)
                                n82 = Not(x=w253) -> (.not. x?=w252:bool)
                                n83 = case shown="False" w252 {
                                tunnel: w258 -> [_ w261]
                                tunnel: [w259 w260] -> w255
                                tunnel: w256 -> [w259 _]
                                frame False {
                                }
                                frame True {
                                n84 = call <vilib>:"Draw Flattened Pixmap.vi"("picture"=w261) -> ("new picture"=w260:picture)  [unwired: 8 in]
                                }
                                }
                                }
                                }
                                n85 = local write "Reagent Pic 2"(w245) -> ()
                              }
                              frame #1 {
                                n86 = Wait (ms)(milliseconds to wait=100) -> ()  [unwired: 1 out]
                              }
                            }
                          }
                          frame #1 {
                            n87 = flat-sequence {
                              tunnel: w264 -> [w270]
                              tunnel: w263 -> [w268]
                              frame #0 {
                                n88 = local read "reagent name 1"() -> (w265:string)
                                n89 = String Length(string=w265) -> (length=w269:i32)
                                n90 = Greater Than 0?(x=w269) -> (x > 0?=w267:bool)
                                n91 = case shown="True" w267 {
                                tunnel: w270 -> [_ w276]
                                tunnel: w268 -> [w271 _]
                                tunnel: [w271 w275] -> w266
                                tunnel: w265 -> [_ w274]
                                frame False {
                                }
                                frame True {
                                n92 = call "Image_from_name.vi"("Chemical Name"=w274) -> ("error out"=w277:errorcluster, "Downloaded Picture"=w278:picture)  [unwired: 8 in, 1 out]
                                n93 = Unbundle By Name(w277) -> ("status"=w273:bool)
                                n94 = Not(x=w273) -> (.not. x?=w272:bool)
                                n95 = case shown="True" w272 {
                                tunnel: w278 -> [_ w281]
                                tunnel: [w279 w280] -> w275
                                tunnel: w276 -> [w279 _]
                                frame False {
                                }
                                frame True {
                                n96 = call <vilib>:"Draw Flattened Pixmap.vi"("picture"=w281) -> ("new picture"=w280:picture)  [unwired: 8 in]
                                }
                                }
                                }
                                }
                                n97 = local write "Reagent Pic 1"(w266) -> ()
                              }
                              frame #1 {
                                n98 = Wait (ms)(milliseconds to wait=100) -> ()  [unwired: 1 out]
                              }
                            }
                          }
                          frame #2 {
                            n99 = flat-sequence {
                              tunnel: w284 -> [w290]
                              tunnel: w283 -> [w288]
                              frame #0 {
                                n100 = local read "Product name"() -> (w285:string)
                                n101 = String Length(string=w285) -> (length=w289:i32)
                                n102 = Greater Than 0?(x=w289) -> (x > 0?=w287:bool)
                                n103 = case shown="True" w287 {
                                tunnel: w290 -> [_ w296]
                                tunnel: w288 -> [w291 _]
                                tunnel: [w291 w295] -> w286
                                tunnel: w285 -> [_ w294]
                                frame False {
                                }
                                frame True {
                                n104 = call "Image_from_name.vi"("Chemical Name"=w294) -> ("error out"=w297:errorcluster, "Downloaded Picture"=w298:picture)  [unwired: 8 in, 1 out]
                                n105 = Unbundle By Name(w297) -> ("status"=w292:bool)
                                n106 = Not(x=w292) -> (.not. x?=w293:bool)
                                n107 = case shown="False" w293 {
                                tunnel: w298 -> [_ w301]
                                tunnel: [w299 w300] -> w295
                                tunnel: w296 -> [w299 _]
                                frame False {
                                }
                                frame True {
                                n108 = call <vilib>:"Draw Flattened Pixmap.vi"("picture"=w301) -> ("new picture"=w300:picture)  [unwired: 8 in]
                                }
                                }
                                }
                                }
                                n109 = local write "Product Pic"(w286) -> ()
                              }
                              frame #1 {
                                n110 = Wait (ms)(milliseconds to wait=100) -> ()  [unwired: 1 out]
                              }
                            }
                          }
                          frame #3 {
                            n111 = flat-sequence {
                              tunnel: w304 -> [w310]
                              tunnel: w303 -> [w308]
                              frame #0 {
                                n112 = local read "reagent name 6"() -> (w305:string)
                                n113 = String Length(string=w305) -> (length=w309:i32)
                                n114 = Greater Than 0?(x=w309) -> (x > 0?=w307:bool)
                                n115 = case shown="True" w307 {
                                tunnel: w310 -> [_ w316]
                                tunnel: w308 -> [w311 _]
                                tunnel: [w311 w315] -> w306
                                tunnel: w305 -> [_ w314]
                                frame False {
                                }
                                frame True {
                                n116 = call "Image_from_name.vi"("Chemical Name"=w314) -> ("error out"=w317:errorcluster, "Downloaded Picture"=w318:picture)  [unwired: 8 in, 1 out]
                                n117 = Unbundle By Name(w317) -> ("status"=w312:bool)
                                n118 = Not(x=w312) -> (.not. x?=w313:bool)
                                n119 = case shown="False" w313 {
                                tunnel: w318 -> [_ w321]
                                tunnel: [w319 w320] -> w315
                                tunnel: w316 -> [w319 _]
                                frame False {
                                }
                                frame True {
                                n120 = call <vilib>:"Draw Flattened Pixmap.vi"("picture"=w321) -> ("new picture"=w320:picture)  [unwired: 8 in]
                                }
                                }
                                }
                                }
                                n121 = local write "Reagent Pic 6"(w306) -> ()
                              }
                              frame #1 {
                                n122 = Wait (ms)(milliseconds to wait=100) -> ()  [unwired: 1 out]
                              }
                            }
                          }
                          frame #4 {
                            n123 = flat-sequence {
                              tunnel: w324 -> [w330]
                              tunnel: w323 -> [w328]
                              frame #0 {
                                n124 = local read "reagent name 5"() -> (w325:string)
                                n125 = String Length(string=w325) -> (length=w329:i32)
                                n126 = Greater Than 0?(x=w329) -> (x > 0?=w327:bool)
                                n127 = case shown="True" w327 {
                                tunnel: w330 -> [_ w336]
                                tunnel: w328 -> [w331 _]
                                tunnel: [w331 w335] -> w326
                                tunnel: w325 -> [_ w334]
                                frame False {
                                }
                                frame True {
                                n128 = call "Image_from_name.vi"("Chemical Name"=w334) -> ("error out"=w337:errorcluster, "Downloaded Picture"=w338:picture)  [unwired: 8 in, 1 out]
                                n129 = Unbundle By Name(w337) -> ("status"=w332:bool)
                                n130 = Not(x=w332) -> (.not. x?=w333:bool)
                                n131 = case shown="False" w333 {
                                tunnel: w338 -> [_ w341]
                                tunnel: [w339 w340] -> w335
                                tunnel: w336 -> [w339 _]
                                frame False {
                                }
                                frame True {
                                n132 = call <vilib>:"Draw Flattened Pixmap.vi"("picture"=w341) -> ("new picture"=w340:picture)  [unwired: 8 in]
                                }
                                }
                                }
                                }
                                n133 = local write "Reagent pic 5"(w326) -> ()
                              }
                              frame #1 {
                                n134 = Wait (ms)(milliseconds to wait=100) -> ()  [unwired: 1 out]
                              }
                            }
                          }
                          frame #5 {
                            n135 = flat-sequence {
                              tunnel: w344 -> [w348]
                              tunnel: w343 -> [w347]
                              frame #0 {
                                n136 = local read "reagent name 4"() -> (w345:string)
                                n137 = String Length(string=w345) -> (length=w350:i32)
                                n138 = Greater Than 0?(x=w350) -> (x > 0?=w349:bool)
                                n139 = case shown="True" w349 {
                                tunnel: w347 -> [_ w356]
                                tunnel: w348 -> [w351 _]
                                tunnel: [w351 w355] -> w346
                                tunnel: w345 -> [_ w354]
                                frame False {
                                }
                                frame True {
                                n140 = call "Image_from_name.vi"("Chemical Name"=w354) -> ("error out"=w357:errorcluster, "Downloaded Picture"=w358:picture)  [unwired: 8 in, 1 out]
                                n141 = Unbundle By Name(w357) -> ("status"=w352:bool)
                                n142 = Not(x=w352) -> (.not. x?=w353:bool)
                                n143 = case shown="False" w353 {
                                tunnel: w358 -> [_ w361]
                                tunnel: [w359 w360] -> w355
                                tunnel: w356 -> [w359 _]
                                frame False {
                                }
                                frame True {
                                n144 = call <vilib>:"Draw Flattened Pixmap.vi"("picture"=w361) -> ("new picture"=w360:picture)  [unwired: 8 in]
                                }
                                }
                                }
                                }
                                n145 = local write "Reagent Pic 4"(w346) -> ()
                              }
                              frame #1 {
                                n146 = Wait (ms)(milliseconds to wait=100) -> ()  [unwired: 1 out]
                              }
                            }
                          }
                          frame #6 {
                            n147 = flat-sequence {
                              tunnel: w364 -> [w368]
                              tunnel: w363 -> [w367]
                              frame #0 {
                                n148 = local read "reagent  name 3"() -> (w365:string)
                                n149 = String Length(string=w365) -> (length=w370:i32)
                                n150 = Greater Than 0?(x=w370) -> (x > 0?=w369:bool)
                                n151 = case shown="True" w369 {
                                tunnel: w367 -> [_ w376]
                                tunnel: w368 -> [w371 _]
                                tunnel: [w371 w375] -> w366
                                tunnel: w365 -> [_ w374]
                                frame False {
                                }
                                frame True {
                                n152 = call "Image_from_name.vi"("Chemical Name"=w374) -> ("error out"=w377:errorcluster, "Downloaded Picture"=w378:picture)  [unwired: 8 in, 1 out]
                                n153 = Unbundle By Name(w377) -> ("status"=w372:bool)
                                n154 = Not(x=w372) -> (.not. x?=w373:bool)
                                n155 = case shown="False" w373 {
                                tunnel: w378 -> [_ w381]
                                tunnel: [w379 w380] -> w375
                                tunnel: w376 -> [w379 _]
                                frame False {
                                }
                                frame True {
                                n156 = call <vilib>:"Draw Flattened Pixmap.vi"("picture"=w381) -> ("new picture"=w380:picture)  [unwired: 8 in]
                                }
                                }
                                }
                                }
                                n157 = local write "Reagent Pic 3"(w366) -> ()
                              }
                              frame #1 {
                                n158 = Wait (ms)(milliseconds to wait=100) -> ()  [unwired: 1 out]
                              }
                            }
                          }
                        }
                      }
                      frame #3 {
                        n159 = local read "BAY 1"() -> (w393:u16)
                        n160 = local read "BAY 2"() -> (w392:u16)
                        n161 = local read "BAY 3"() -> (w391:u16)
                        n162 = local read "BAY 4"() -> (w390:u16)
                        n163 = local read "BAY 5"() -> (w389:u16)
                        n164 = local read "tube_id(in)"() -> (w400:enum16{".01", ".02", ".03", ".04"}[])
                        n165 = local read "Vr4"() -> (w403:dbl)
                        n166 = local read "tube_length(in)"() -> (w401:dbl[])
                        n167 = Build Array(w393, w392, w391, w390, w389) -> (w388:u16[])
                        n168 = local read "Vr3"() -> (w404:dbl)
                        n169 = local read "new_reactor_length"() -> (w398:bool[])
                        n170 = local read "Vr1"() -> (w406:dbl)
                        n171 = local read "Vr5"() -> (w402:dbl)
                        n172 = local read "Vr2"() -> (w405:dbl)
                        n173 = local read "new_reactor_volume"() -> (w396:bool[])
                        n174 = for {
                          N: 5 -> [_]
                          tunnel: w396 -> [w410] mode=indexing
                          tunnel: [w407] -> w394 mode=indexing
                          n175 = Select(t=1.0, s=w410, f=0.0) -> (s? t:f=w407:dbl)
                        }
                        n176 = for {
                          N: 5 -> [_]
                          tunnel: w398 -> [w414] mode=indexing
                          tunnel: [w411] -> w397 mode=indexing
                          n177 = Select(t=1.0, s=w414, f=0.0) -> (s? t:f=w411:dbl)
                        }
                        n178 = script code="tube_diameters = [.01,.02,.03,.04];\naddpath('C:\\Users\\HPLC\\Dropbox (MIT)\\MoD Files\\MATLAB');\ncalculate_reactor_volumes;"("BayConfig"=w388, "Vr1"=w406, "Vr2"=w405, "Vr3"=w404, "Vr4"=w403, "Vr5"=w402, "tube_length"=w401, "tube_id"=w400, "new_len_react"=w397, "new_vol_react"=w394) -> ("Vr1"=w387:dbl, "Vr2"=w386:dbl, "Vr3"=w385:dbl, "Vr4"=w384:dbl, "Vr5"=w383:dbl)  [unwired: 1 in, 1 out]
                        n179 = local write "Vr1"(w387) -> ()
                        n180 = local write "Vr2"(w386) -> ()
                        n181 = local write "Vr3"(w385) -> ()
                        n182 = local write "Vr4"(w384) -> ()
                        n183 = local write "Vr5"(w383) -> ()
                      }
                      frame #4 {
                        n184 = local read "Setup Error"() -> (w417:bool)
                        n185 = case shown="True" w417 {
                          tunnel: [TRUE FALSE] -> w415
                          tunnel: ["" "Sytem setup has not been confirmed!"] -> w416
                          frame False {
                          }
                          frame True {
                            n186 = local read "Error Message"() -> (w422:string)
                            n187 = One Button Dialog(message=w422) -> ()  [unwired: 1 in, 1 out]
                          }
                        }
                        n188 = local write "System Confirm Not Clicked"(w416) -> ()
                        n189 = local write "Setup Confirm"(w415) -> ()
                      }
                    }
                  }
                }
              }
            }
            n190 = local read "Stop"() -> (w201:bool)
            n191 = Or(x=w202, y=w201) -> (x .or. y?=w200:bool)
            n192 = disable-structure shown="Disabled" {
              disable-tunnel: 400 -> [w208 _]
              frame Disabled {
                n193 = event shown="[1]" {
                  selector: _ -> [_ _]
                  dyn-events: _ -> [_ _]
                  timeout: w208 -> [_ _]
                  event Timeout {
                    n194 = event-data() -> ()  [unwired: 1 in, 3 out]
                  }
                  event #1 (no event record) {
                    n195 = event-data() -> ()  [unwired: 1 in, 6 out]
                    n196 = local read "Setup Confirm"() -> (w209:bool)
                    n197 = local read "Reaction Scheme Confirm"() -> (w210:bool)
                    n198 = Not(x=w209) -> (.not. x?=w212:bool)
                    n199 = And(x=w210, y=w212) -> (x .and. y?=w211:bool)
                    n200 = case shown="True" w211 {
                      frame False {
                      }
                      frame True {
                        w214 = u16 0 items=["                     Bypass", "                Hot Reactor", "                 Separator"] ("BAY 5")
                        w215 = u16 0 items=["                     Bypass", "                Hot Reactor", "                  Separator"] ("BAY 4")
                        w216 = u16 0 items=["                     Bypass", "                 Hot Reactor", "                  Separator"] ("BAY 3")
                        w217 = u16 0 items=["                     Bypass", "                Hot Reactor", "                  Separator"] ("BAY 2")
                        w218 = u16 0 items=["                 Bypass", "             Hot Reactor", "               Separator"] ("BAY 1")
                        n201 = local write "BAY 3"(w216) -> ()
                        n202 = local write "BAY 4"(w215) -> ()
                        n203 = local write "BAY 5"(w214) -> ()
                        n204 = local write "BAY 2"(w217) -> ()
                        n205 = local write "BAY 1"(w218) -> ()
                        n206 = local write "Synthesis Route Array"(string[][] [["3-Br-Pyridine _ Biphenyl", "K2CO3", "PhB(OH)2", "", "", ""]] ("Synthesis Route Array")) -> ()
                      }
                    }
                  }
                }
              }
              frame Enabled {
              }
            }
            n207 = disable-structure shown="Disabled" {
              disable-tunnel: 400 -> [w204 _]
              frame Disabled {
                n208 = event shown="[1]" {
                  selector: _ -> [_ _]
                  dyn-events: _ -> [_ _]
                  timeout: w204 -> [_ _]
                  event Timeout {
                    n209 = event-data() -> ()  [unwired: 1 in, 3 out]
                  }
                  event #1 (no event record) {
                    n210 = event-data() -> ()  [unwired: 1 in, 6 out]
                    n211 = call "File Dialog"("prompt"="Load previously saved xml file") -> ("selected path"=w206:path)  [unwired: 11 in, 3 out]
                    n212 = Path To String(path=w206) -> (string=w205:string)
                    n213 = script code="xmlDoc = xmlread(file_path);\nroot = xmlDoc.getDocumentElement();\nb = root.getChildNodes;\nrecipe = b.getElementsByTagName('Bay1').item(0);"("file_path"=w205) -> ()  [unwired: 1 in, 1 out]
                  }
                }
              }
              frame Enabled {
              }
            }
          }
        }
        frame #1 {
          n214 = local read "Stop"() -> (w424:bool)
          n215 = Not(x=w424) -> (.not. x?=w423:bool)
          n216 = case shown="True" w423 {
            tunnel: w425 -> [_ w428]
            frame False {
              "stop_button clicked" <- TRUE ("stop_button clicked")
            }
            frame True {
              # "Parameters Initilization"
              n217 = flat-sequence {
                tunnel: w428 -> [w430]
                tunnel: [w429] -> w427
                tunnel: w427 -> [w589]
                frame #0 {
                  # "Setup bays(RFID - verify)"
                  n218 = disable-structure shown="Disabled" {
                    frame Disabled {
                      n219 = local read "BAY 1"() -> ()  [unwired: 1 out]
                      n220 = local read "BAY 2"() -> ()  [unwired: 1 out]
                      n221 = local read "BAY 3"() -> ()  [unwired: 1 out]
                      n222 = local read "BAY 4"() -> ()  [unwired: 1 out]
                      n223 = local read "BAY 5"() -> ()  [unwired: 1 out]
                    }
                    frame Enabled {
                    }
                  }
                }
                frame #1 {
                  n224 = while {
                    tunnel: w430 -> [w433]
                    tunnel: [w432] -> w429
                    stop <- w436 stop-if-true
                    n225 = flat-sequence {
                      tunnel: [w450] -> w432
                      tunnel: w433 -> [w531]
                      tunnel: [w449] -> w431
                      frame #0 {
                        n226 = while {
                          stop <- w440 stop-if-true
                          n227 = event shown="[1] \"System Parameters Confirm Button\": Value Change" {
                            selector: _ -> [_ _]
                            dyn-events: _ -> [_ _]
                            timeout: u32 200 ("milliseconds to wait") -> [_ _]
                            tunnel: [FALSE TRUE] -> w438
                            event Timeout {
                              n228 = event-data() -> ()  [unwired: 1 in, 3 out]
                            }
                            event "System Parameters Confirm Button": Value Change {
                              n229 = event-data() -> ()  [unwired: 1 in, 5 out]
                              n230 = local write "System Parameters Confirm Button"(FALSE) -> ()
                            }
                          }
                          n231 = Wait (ms)(milliseconds to wait=u32 500) -> ()  [unwired: 1 out]
                          n232 = local read "Stop"() -> (w441:bool)
                          n233 = Or(x=w441, y=w438) -> (x .or. y?=w440:bool)
                        }
                      }
                      frame #1 {
                        w470 = 0 ("disabled index (col)")
                        w482 = 1 ("disabled index (col)")
                        # "Do while parameters have not been correctly entered"
                        n234 = local read "Bay Parameters"() -> (w469:T2)
                        n235 = local read "Synthesis Route Array"() -> (w483:string[][])
                        n236 = local read "Total Number of Experiments"() -> (w502:dbl)
                        n237 = Unbundle By Name(w469) -> ("Continue from previous optimization?"=w530:bool)
                        n238 = Unbundle By Name(w469) -> ("Excel File Name"=w532:string)
                        n239 = Unbundle By Name(w469) -> ("Matlab File"=w528:string)
                        n240 = Unbundle By Name(w469) -> ("Bay 1.Run at set flowrate"=w574:bool)
                        n241 = Unbundle By Name(w469) -> ("Bay 1.Pump 1 Flowrate"=w580:dbl)
                        n242 = Unbundle By Name(w469) -> ("Bay 1.Pump 2 Flowrate"=w579:dbl)
                        n243 = Unbundle By Name(w469) -> ("Bay 2.Run at set flowrate"=w572:bool)
                        n244 = Unbundle By Name(w469) -> ("Bay 2.Pump 3 Flowrate"=w578:dbl)
                        n245 = Unbundle By Name(w469) -> ("Bay 3.Pump 4 Flowrate"=w577:dbl)
                        n246 = Unbundle By Name(w469) -> ("Bay 3.Run at set flowrate"=w571:bool)
                        n247 = Unbundle By Name(w469) -> ("Bay 4.Run at set flowrate"=w568:bool)
                        n248 = Unbundle By Name(w469) -> ("Bay 4.Pump 5 Flowrate"=w576:dbl)
                        n249 = Unbundle By Name(w469) -> ("Bay 5.Pump 6 Flowrate"=w575:dbl)
                        n250 = Unbundle By Name(w469) -> ("Bay 5.Run at set flowrate"=w567:bool)
                        n251 = Index Array(array=w483, index (row)=3, index (col)=w482) -> (element=w476:string)
                        n252 = Index Array(array=w483, index (row)=2, index (col)=w482) -> (element=w474:string)
                        n253 = Index Array(array=w483, index (row)=1, index (col)=w482) -> (element=w472:string)
                        n254 = Index Array(array=w483, index (row)=0, index (col)=w482) -> (element=w485:string)
                        n255 = Index Array(array=w483, index (row)=4, index (col)=w482) -> (element=w478:string)
                        n256 = Index Array(array=w483, index (row)=5, index (col)=w482) -> (element=w480:string)
                        n257 = Build Array(w485, w472, w474, w476, w478, w480) -> (w486:string[])
                        n258 = Index Array(array=w483, index (row)=0 ("index"), index (col)=w470) -> (element=w508:string)
                        n259 = for {
                          tunnel: w486 -> [w582] mode=indexing
                          tunnel: [w581] -> w471 mode=indexing
                          n260 = script code="ctemp1 = str2num(c_temp);"("c_temp"=w582) -> ("ctemp1"=w581:dbl)  [unwired: 1 in, 1 out]
                        }
                        n261 = Boolean To (0,1)(Boolean=w572) -> (0, 1=w527:i16)
                        n262 = Boolean To (0,1)(Boolean=w568) -> (0, 1=w569:i16)
                        n263 = Boolean To (0,1)(Boolean=w571) -> (0, 1=w570:i16)
                        n264 = Boolean To (0,1)(Boolean=w530) -> (0, 1=w529:i16)
                        n265 = Boolean To (0,1)(Boolean=w574) -> (0, 1=w573:i16)
                        n266 = Boolean To (0,1)(Boolean=w567) -> (0, 1=w566:i16)
                        n267 = Index Array(array=w483, index (row)=1 ("index"), index (col)=w470) -> (element=w503:string)
                        n268 = Index Array(array=w483, index (row)=2 ("index"), index (col)=w470) -> (element=w504:string)
                        n269 = Unbundle By Name(w469) -> ("Bay 1.optimize_temp"=w565:bool)
                        n270 = Unbundle By Name(w469) -> ("Bay 1.optimize_tau"=w563:bool)
                        n271 = Unbundle By Name(w469) -> ("Bay 2.optimize_temp"=w561:bool)
                        n272 = Unbundle By Name(w469) -> ("Bay 2.optimize_tau"=w559:bool)
                        n273 = Unbundle By Name(w469) -> ("Bay 3.optimize_temp"=w557:bool)
                        n274 = Unbundle By Name(w469) -> ("Bay 3.optimize_tau"=w555:bool)
                        n275 = Unbundle By Name(w469) -> ("Bay 4.optimize_temp"=w553:bool)
                        n276 = Unbundle By Name(w469) -> ("Bay 4.optimize_tau"=w551:bool)
                        n277 = Index Array(array=w483, index (row)=3 ("index"), index (col)=w470) -> (element=w505:string)
                        n278 = Boolean To (0,1)(Boolean=w553) -> (0, 1=w552:i16)
                        n279 = Boolean To (0,1)(Boolean=w551) -> (0, 1=w550:i16)
                        n280 = Index Array(array=w483, index (row)=4 ("index"), index (col)=w470) -> (element=w506:string)
                        n281 = Boolean To (0,1)(Boolean=w555) -> (0, 1=w554:i16)
                        n282 = Boolean To (0,1)(Boolean=w561) -> (0, 1=w560:i16)
                        n283 = Boolean To (0,1)(Boolean=w565) -> (0, 1=w564:i16)
                        n284 = Boolean To (0,1)(Boolean=w559) -> (0, 1=w558:i16)
                        n285 = Boolean To (0,1)(Boolean=w563) -> (0, 1=w562:i16)
                        n286 = Boolean To (0,1)(Boolean=w557) -> (0, 1=w556:i16)
                        n287 = Unbundle By Name(w469) -> ("Bay 5.optimize_temp"=w549:bool)
                        n288 = Unbundle By Name(w469) -> ("Bay 5.optimize_tau"=w547:bool)
                        n289 = Index Array(array=w483, index (row)=5 ("index"), index (col)=w470) -> (element=w507:string)
                        n290 = Boolean To (0,1)(Boolean=w549) -> (0, 1=w548:i16)
                        n291 = Boolean To (0,1)(Boolean=w547) -> (0, 1=w546:i16)
                        n292 = Build Array(w564, w562, w560, w558, w556, w554, w552, w550, w548, w546) -> (w545:i16[])
                        n293 = Unbundle By Name(w469) -> ("Bay 1.Temperature Params"=w542:dbl[])
                        n294 = Unbundle By Name(w469) -> ("Bay 2.Temperature Params"=w541:dbl[])
                        n295 = Unbundle By Name(w469) -> ("Bay 2.Resisdence time params"=w536:dbl[])
                        n296 = Unbundle By Name(w469) -> ("Bay 3.Temperature Params"=w540:dbl[])
                        n297 = Unbundle By Name(w469) -> ("Bay 3.Resisdence time params"=w535:dbl[])
                        n298 = Unbundle By Name(w469) -> ("Bay 4.Temperature Params"=w539:dbl[])
                        n299 = Unbundle By Name(w469) -> ("Bay 4.Resisdence time params"=w534:dbl[])
                        n300 = Unbundle By Name(w469) -> ("Bay 5.Temperature Params"=w538:dbl[])
                        n301 = Unbundle By Name(w469) -> ("Bay 5.Resisdence time params"=w533:dbl[])
                        n302 = Unbundle By Name(w469) -> ("Bay 1.pump params 2"=w501:dbl[])
                        n303 = Unbundle By Name(w469) -> ("Bay 1.pump params 1"=w537:dbl[])
                        n304 = Unbundle By Name(w469) -> ("Bay 1.Run at set temperature"=w492:bool)
                        n305 = Unbundle By Name(w469) -> ("Bay 2.Run at set temperature"=w490:bool)
                        n306 = Unbundle By Name(w469) -> ("Bay 3.Run at set temperature"=w489:bool)
                        n307 = Unbundle By Name(w469) -> ("Bay 4.Run at set temperature"=w488:bool)
                        n308 = Unbundle By Name(w469) -> ("Bay 5.Run at set temperature"=w487:bool)
                        n309 = Unbundle By Name(w469) -> ("Bay 3.Temperature"=w498:dbl)
                        n310 = Unbundle By Name(w469) -> ("Bay 1.Temperature"=w500:dbl)
                        n311 = Unbundle By Name(w469) -> ("Bay 2.Temperature"=w499:dbl)
                        n312 = Unbundle By Name(w469) -> ("Bay 4.Temperature"=w497:dbl)
                        n313 = Unbundle By Name(w469) -> ("Bay 5.Temperature"=w496:dbl)
                        n314 = Unbundle By Name(w469) -> ("Bay 3.pump_num_ratio"=w521:dbl)
                        n315 = Unbundle By Name(w469) -> ("Bay 4.pump_num_ratio"=w518:dbl)
                        n316 = Unbundle By Name(w469) -> ("Bay 5.pump_num_ratio"=w515:dbl)
                        n317 = Unbundle By Name(w469) -> ("Bay 2.pump_num_ratio"=w524:dbl)
                        n318 = Unbundle By Name(w469) -> ("Bay 4.pump_at_ratio"=w520:bool)
                        n319 = Boolean To (0,1)(Boolean=w520) -> (0, 1=w519:i16)
                        n320 = Unbundle By Name(w469) -> ("Bay 3.pump_at_ratio"=w523:bool)
                        n321 = Boolean To (0,1)(Boolean=w523) -> (0, 1=w522:i16)
                        n322 = Unbundle By Name(w469) -> ("Bay 5.pump_at_ratio"=w517:bool)
                        n323 = Boolean To (0,1)(Boolean=w517) -> (0, 1=w516:i16)
                        n324 = Unbundle By Name(w469) -> ("Bay 2.pump_at_ratio"=w526:bool)
                        n325 = Boolean To (0,1)(Boolean=w526) -> (0, 1=w525:i16)
                        n326 = Build Array(w500, w499, w498, w497, w496) -> (w495:dbl[])
                        n327 = Build Array(w492, w490, w489, w488, w487) -> (w491:bool[])
                        n328 = local read "Syringe_pump?"() -> (w448:bool)
                        n329 = for {
                          N: 5 -> [_]
                          tunnel: w491 -> [w586] mode=indexing
                          tunnel: [w585] -> w493 mode=indexing
                          n330 = Select(t=1.0, s=w586, f=0.0) -> (s? t:f=w585:dbl)
                        }
                        n331 = Unbundle By Name(w469) -> ("Internal Standard?"=w460:bool)
                        n332 = Unbundle By Name(w469) -> ("increas_decrease_hplc_peak"=w461:bool)
                        n333 = Unbundle By Name(w469) -> ("Hplc Wait time(min)"=w453:dbl)
                        n334 = Unbundle By Name(w469) -> ("Total Number of Experiments 2"=w452:dbl)
                        n335 = Unbundle By Name(w469) -> ("hplc_start"=w457:dbl)
                        n336 = Unbundle By Name(w469) -> ("ISTD start"=w455:dbl)
                        n337 = Unbundle By Name(w469) -> ("hplc_end"=w456:dbl)
                        n338 = Unbundle By Name(w469) -> ("throughput_yield"=w462:bool)
                        n339 = Unbundle By Name(w469) -> ("ISTD end"=w454:dbl)
                        n340 = Select(t=1.0, s=w448, f=0.0) -> (s? t:f=w447:dbl)
                        n341 = Select(t=1.0, s=w461, f=0.0) -> (s? t:f=w459:dbl)
                        n342 = Select(t=1.0, s=w460, f=0.0) -> (s? t:f=w458:dbl)
                        n343 = Select(t=0.0, s=w462, f=1.0) -> (s? t:f=w451:dbl)
                        n344 = script code="system_error = 0;\nnumPeaks = 1;\nstart_phase_time = 1;\nis_redo_exp = 0;\nFvalues = [];\nHPLC_Area = [];\n\nT1_span = [1 1]; T2_span = [1 1]; T3_span = [1 1]; T4_span = [1 1]; T5_span = [1 1];\nT_span = [T1_span;T2_span;T3_span;T4_span;T5_span];\n p1_span =  [1 1]; p2_span =  [1 1]; p3_span =  [1 1]; p4_span =  [1 1]; p5_span =  [1 1];  p6_span =  [1 1];\nOpt_params = [0 0 0 0 0 0 0 0 0 0 0];\nT_params = [T1_params;T2_params;T3_params;T4_params;T5_params];\npump_params = [pump1_params;pump2_params;pump3_params;pump4_params;pump5_params;pump6_params];\nopt_ctr = 0;ncall = 100;record_data = true;\nT1_SP = 23; T2_SP = 23; T3_SP = 23; T4_SP = 23; T5_SP = 23;\nT_span = [T1_span;T2_span;T3_span;T4_span;T5_span];\np_span = [p1_span;p2_span;p3_span;p4_span;p5_span;p6_span];\nno_errors = 1;\nP1 = 0; P2 =0; P3 = 0; P4 = 0; P5 = 0; P6 = 0;\nP = [P1, P2, P3,P4, P5, P6];\nis_first_set_of_exp = true;\nerror_message = 'System has no errors to report';\naddpath(genpath('C:\\Users\\HPLC\\Dropbox (MIT)\\MoD Files\\MATLAB'))\n%addpath(genpath('C:\\Users\\Admin\\Dropbox (MIT)\\MoD Files\\MATLAB'))\nallMSData = [];allHPLCData = [];allHPLCFile = [];\nBay_ratio = [0,Bay2_ratio,Bay3_ratio,Bay4_ratio,Bay5_ratio];\nBay_pump_ratio = [1, Bay2_pump_ratio, Bay3_pump_ratio, Bay4_pump_ratio, Bay5_pump_ratio];\nP_setrate = [P1_setrate, P2_setrate, P3_setrate, P4_setrate, P5_setrate, P6_setrate];\nuse_flowrate = [use_flowrate1, use_flowrate2,use_flowrate3, use_flowrate4, use_flowrate5];\npump_chem_name= []\nCurrExp = 1;\n% ****************************************************************************************************\n%Setup optimization\n   setup_optimization_params;\n   initialize_opt = 0;\n   nstop0 = 0;\n%*****************************************************************************************************\n% Setup excel and xml file writing\npath(path, pa);\nnumMSSig = 1;\nsetup_excel_output;\n%***************************************************************************************************\nredo = false;\nncall = ncall_in;"("use_flowrate1"=w573, "P1_setrate"=w580, "P2_setrate"=w579, "P3_setrate"=w578, "P4_setrate"=w577, "P5_setrate"=w576, "P6_setrate"=w575, "use_flowrate2"=w527, "use_flowrate3"=w570, "use_flowrate4"=w569, "use_flowrate5"=w566, "Optimize_params"=w545, "T1_params"=w542, "T2_params"=w541, "T3_params"=w540, "T4_params"=w539, "T5_params"=w538, "pump1_params"=w537, "pump3_params"=w536, "pump4_params"=w535, "pump5_params"=w534, "pump6_params"=w533, "xl_file"=w532, "pa"=w531, "Continue"=w529, "matlabsavefile"=w528, "Bay2_ratio"=w525, "Bay2_pump_ratio"=w524, "Bay3_ratio"=w522, "Bay3_pump_ratio"=w521, "Bay4_ratio"=w519, "Bay4_pump_ratio"=w518, "Bay5_ratio"=w516, "Bay5_pump_ratio"=w515, "pump1_chem"=w508, "pump6_chem"=w507, "pump5_chem"=w506, "pump4_chem"=w505, "pump3_chem"=w504, "pump2_chem"=w503, "Pump_concen"=w471, "ncall_in"=w502, "pump2_params"=w501, "T_SP"=w495, "Run_at_T_SP"=w493, "dcr_hplc_peak"=w459, "use_internal_std"=w458, "hplc_peak_start"=w457, "hplc_peak_end"=w456, "ISTD_start"=w455, "ISTD_end"=w454, "hplc_wait_time"=w453, "tot_num_exp"=w452, "throughput_yield"=w451, "syringe_pump"=w447) -> ("no_errors"=w544:dbl, "error_message"=w543:string)  [unwired: 1 in, 1 out]
                        n345 = Not Equal To 0?(x=w544) -> (x != 0?=w449:bool)
                        n346 = Not(x=w449) -> (.not. x?=w450:bool)
                        n347 = case shown="False" w450 {
                          tunnel: w543 -> [_ w588]
                          frame False {
                            n348 = local write "Setup Confirm 2"(TRUE ("Setup Confirm 2")) -> ()
                          }
                          frame True {
                            n349 = One Button Dialog(message=w588) -> ()  [unwired: 1 in, 1 out]
                          }
                        }
                      }
                    }
                    n350 = local read "Stop"() -> (w435:bool)
                    n351 = Or(x=w431, y=w435) -> (x .or. y?=w436:bool)
                    n352 = Wait (ms)(milliseconds to wait=u32 500) -> ()  [unwired: 1 out]
                  }
                }
                frame #2 {
                  n353 = local write "System Error"(w589) -> ()
                }
              }
            }
          }
        }
        frame #2 {
          # "Run Initial diagnostics"
        }
        frame #3 {
          # "Run System"
          n354 = while {
            tunnel: w590 -> [w1307]
            stop <- w1311 stop-if-true
            n355 = local read "running?"() -> (w1306:bool)
            n356 = local read "Temperature Control 1"() -> (w1308:bool)
            n357 = And(x=w1306, y=w1308) -> (x .and. y?=w1309:bool)
            n358 = case shown="True" w1309 {
              tunnel: w1307 -> [_ w1313]
              frame False {
                n359 = local write "Temp SS? 1"(TRUE ("Temp SS? 1")) -> ()
              }
              frame True {
                # "Bay 1 Temperature Controller"
                n360 = local read "Temperature SP 1"() -> (w1314:dbl)
                n361 = local read "Temperature 1"() -> (w1318:dbl)
                n362 = local read "SSR Duration 1"() -> (w1333:dbl)
                n363 = call-poly <vilib>:"PID Online Autotuning.vi"("setpoint"=w1314, "manipulated variable"=w1333, "autotuning parameters"=T9 {"type of controller"=enum."PID", "relay cycles"=3, "relay amplitude"=1.0, "control specifications"=enum."Normal", "PV noise level"=0.1} ("Autotuning Parameters R1"), "process variable"=w1318, "PID gains in"=T8 {"Proportional gain Kc"=0.38538, "Integral time Ti (sec)"=0.524375, "Derivative time Ti (sec)"=0.12585} ("PID gains 2")) -> ("setpoint out"=w1339:dbl, "process variable out"=w1338:dbl, "PID gains out"=w1335:T17)  [unwired: 6 in, 2 out]
                n364 = call <vilib>:"PID Autotuning (Temperature).vi"("desired temperature"=w1339, "measured temperature"=w1338, "plant parameters in"=w1335, "output range"=cluster{"output high":dbl, "output low":dbl} {"output high"=3.0, "output low"=-1.0} ("Output range")) -> ("output"=w1331:dbl)  [unwired: 12 in, 3 out]
                n365 = local write "SSR Duration 1"(w1331) -> ()
                n366 = Subtract(x=w1314, y=w1318) -> (x-y=w1325:dbl)
                n367 = Absolute Value(x=w1325) -> (abs(x)=w1328:dbl)
                n368 = Multiply(x=1000.0, y=w1331) -> (x*y=w1329:dbl)
                n369 = Greater Than 0?(x=w1329) -> (x > 0?=w1323:bool)
                n370 = Less Or Equal?(x=w1328, y=1.2) -> (x <= y?=w1326:bool)
                n371 = Greater?(x=w1314, y=w1318) -> (0:w1324:bool)
                n372 = And(x=w1323, y=w1324) -> (x .and. y?=w1321:bool)
                n373 = local write "Temp SS? 1"(w1326) -> ()
                n374 = Subtract(x=w1318, y=10.0) -> (x-y=w1319:dbl)
                n375 = Less?(x=w1319, y=w1314) -> (x < y?=w1322:bool)
                n376 = And(x=w1322, y=w1321) -> (x .and. y?=w1320:bool)
                n377 = case shown="True" w1320 {
                  tunnel: [errorcluster {"status"=FALSE, "code"=0, "source"=""} ("error out") w1349] -> _
                  tunnel: 2 -> [_ w1346]
                  tunnel: w1329 -> [w1343 w1347]
                  tunnel: [0.0 w1351] -> w1316
                  tunnel: w1314 -> [_ w1350]
                  tunnel: w1313 -> [_ w1348]
                  frame False {
                    n378 = Absolute Value(x=w1343) -> (abs(x)=w1344:dbl)
                    n379 = Wait (ms)(milliseconds to wait=w1344) -> ()  [unwired: 1 out]
                  }
                  frame True {
                    n380 = call "TurnOnRelayArduino.vi"("channel"=w1346, "duration"=w1347, "LINX Resource"=w1348) -> ("error out"=w1349:errorcluster)  [unwired: 7 in, 1 out]
                    n381 = script code="tempdiff1= SP1 - T1;\nif tempdiff1 > 10\n  if slope1 < .01\n     temp_check1 = temp_check1 + 1;\n  else\n      temp_check1 =0;\n  end\nend\n\nif temp_check1 > 9\n  temp_error1 = 1\nend"("SP1"=w1350) -> ("temp_error1"=w1351:dbl)  [unwired: 1 in, 1 out]
                  }
                }
                n382 = Not Equal To 0?(x=w1316) -> (x != 0?=w1315:bool)
                n383 = case shown="True" w1315 {
                  frame False {
                  }
                  frame True {
                    n384 = local write "Error Message"("Bay 1 Temperature Heating Error") -> ()
                  }
                }
                n385 = case shown="True" w1315 {
                  tunnel: w1315 -> [_ w1341]
                  frame False {
                  }
                  frame True {
                    n386 = local write "System Error"(w1341) -> ()
                    n387 = local write "Stop"(w1341) -> ()
                  }
                }
              }
            }
            n388 = Wait (ms)(milliseconds to wait=u32 400) -> ()  [unwired: 1 out]
            n389 = local read "Stop"() -> (w1311:bool)
          }
          n390 = local read "Bay Parameters"() -> (w594:T2)
          n391 = while {
            tunnel: w590 -> [w1261]
            stop <- w1265 stop-if-true
            n392 = local read "running?"() -> (w1260:bool)
            n393 = local read "Temperature Control 2"() -> (w1262:bool)
            n394 = And(x=w1260, y=w1262) -> (x .and. y?=w1263:bool)
            n395 = case shown="True" w1263 {
              tunnel: w1261 -> [_ w1267]
              frame False {
                n396 = local write "Temp SS? 2"(TRUE ("Temp SS? 2")) -> ()
              }
              frame True {
                # "Bay 2 Temperature Controller"
                n397 = local read "Temperature SP 2"() -> (w1269:dbl)
                n398 = local read "Temperature 2"() -> (w1272:dbl)
                n399 = local read "SSR Duration 2"() -> (w1290:dbl)
                n400 = call-poly <vilib>:"PID Online Autotuning.vi"("setpoint"=w1269, "manipulated variable"=w1290, "autotuning parameters"=T9 {"type of controller"=enum."PID", "relay cycles"=3, "relay amplitude"=1.0, "control specifications"=enum."Normal", "PV noise level"=0.1} ("Autotuning Parameters R1"), "process variable"=w1272, "PID gains in"=T8 {"Proportional gain Kc"=0.38538, "Integral time Ti (sec)"=0.524375, "Derivative time Ti (sec)"=0.12585} ("PID gains 2")) -> ("setpoint out"=w1288:dbl, "process variable out"=w1287:dbl, "PID gains out"=w1293:T17)  [unwired: 6 in, 2 out]
                n401 = call <vilib>:"PID Autotuning (Temperature).vi"("desired temperature"=w1288, "measured temperature"=w1287, "plant parameters in"=w1293, "output range"=cluster{"output high":dbl, "output low":dbl} {"output high"=3.0, "output low"=-1.0} ("Output range")) -> ("output"=w1283:dbl)  [unwired: 12 in, 3 out]
                n402 = local write "SSR Duration 2"(w1283) -> ()
                n403 = Greater?(x=w1269, y=w1272) -> (0:w1278:bool)
                n404 = Multiply(x=1000.0, y=w1283) -> (x*y=w1285:dbl)
                n405 = Greater Than 0?(x=w1285) -> (x > 0?=w1277:bool)
                n406 = And(x=w1277, y=w1278) -> (x .and. y?=w1275:bool)
                n407 = Subtract(x=w1269, y=w1272) -> (x-y=w1280:dbl)
                n408 = Absolute Value(x=w1280) -> (abs(x)=w1282:dbl)
                n409 = Subtract(x=w1272, y=10.0) -> (x-y=w1274:dbl)
                n410 = Less Or Equal?(x=w1282, y=1.2) -> (x <= y?=w1279:bool)
                n411 = local write "Temp SS? 2"(w1279) -> ()
                n412 = Less?(x=w1274, y=w1269) -> (x < y?=w1276:bool)
                n413 = And(x=w1276, y=w1275) -> (x .and. y?=w1271:bool)
                n414 = case shown="True" w1271 {
                  tunnel: [errorcluster {"status"=FALSE, "code"=0, "source"=""} ("error out") w1303] -> _
                  tunnel: 3 -> [_ w1300]
                  tunnel: w1285 -> [w1297 w1301]
                  tunnel: [0.0 w1305] -> w1270
                  tunnel: w1269 -> [_ w1304]
                  tunnel: w1267 -> [_ w1302]
                  frame False {
                    n415 = Absolute Value(x=w1297) -> (abs(x)=w1298:dbl)
                    n416 = Wait (ms)(milliseconds to wait=w1298) -> ()  [unwired: 1 out]
                  }
                  frame True {
                    n417 = call "TurnOnRelayArduino.vi"("channel"=w1300, "duration"=w1301, "LINX Resource"=w1302) -> ("error out"=w1303:errorcluster)  [unwired: 7 in, 1 out]
                    n418 = script code="tempdiff2= SP2 - T2;\nif tempdiff2 > 10\n  if slope2 < .01\n     temp_check2 = temp_check2 + 1;\n  else\n      temp_check2 =0;\n  end\nend\n\nif temp_check2 > 9\n  temp_error2 = 1\nend"("SP2"=w1304) -> ("temp_error2"=w1305:dbl)  [unwired: 1 in, 1 out]
                  }
                }
                n419 = Not Equal To 0?(x=w1270) -> (x != 0?=w1268:bool)
                n420 = case shown="True" w1268 {
                  frame False {
                  }
                  frame True {
                    n421 = local write "Error Message"("Bay 2 Temperature Heating Error") -> ()
                  }
                }
                n422 = case shown="True" w1268 {
                  tunnel: w1268 -> [_ w1295]
                  frame False {
                  }
                  frame True {
                    n423 = local write "Stop"(w1295) -> ()
                    n424 = local write "System Error"(w1295) -> ()
                  }
                }
              }
            }
            n425 = local read "Stop"() -> (w1265:bool)
            n426 = Wait (ms)(milliseconds to wait=u32 400) -> ()  [unwired: 1 out]
          }
          n427 = local read "Stop"() -> (w591:bool)
          n428 = Not(x=w591) -> (.not. x?=w593:bool)
          n429 = case shown="True" w593 {
            tunnel: w594 -> [_ w599]
            tunnel: w592 -> [_ w598]
            tunnel: w590 -> [_ w597]
            frame False {
            }
            frame True {
              n430 = while {
                tunnel: w599 -> [w613]
                tunnel: w598 -> [w605]
                tunnel: w597 -> [w600]
                i -> [w612]
                stop <- w606 stop-if-true
                n431 = local read "running?"() -> (w601:bool)
                n432 = Wait (ms)(milliseconds to wait=u32 1000) -> ()  [unwired: 1 out]
                n433 = Increment(x=w612) -> (x+1=w602:i32)
                n434 = case shown="True" w601 {
                  tunnel: w612 -> [w618 _]
                  tunnel: w613 -> [_ _]
                  tunnel: [w620 w624] -> w603
                  tunnel: [0.0 w625] -> w608
                  tunnel: w605 -> [_ w623]
                  tunnel: w600 -> [_ w621]
                  frame False {
                    # "STANDBY MODE"
                    n435 = Add(x=w618, y=2.0) -> (x+y=w620:dbl)
                  }
                  frame True {
                    n436 = flat-sequence {
                      tunnel: w623 -> [w627]
                      tunnel: [w627] -> w622
                      tunnel: [w637] -> w625
                      tunnel: [200.0] -> w624
                      tunnel: w622 -> [w635]
                      tunnel: w621 -> [w629]
                      frame #0 {
                        n437 = local write "stop_xl_write"(FALSE ("stop_xl_write")) -> ()
                      }
                      frame #1 {
                        # "Increase flowrate of dilution stream"
                        # "Wait mixed stream reaches SL"
                        # "SNOBFIT"
                        # "Optimize"
                        # "Run Experimental Conditions"
                        # "Optimize/Synthesize"
                        n438 = local read "Syringe_pump?"() -> (w628:bool)
                        n439 = local read "Stop"() -> (w632:bool)
                        n440 = Not(x=w632) -> (.not. x?=w631:bool)
                        n441 = case shown="True" w631 {
                          tunnel: [1.0 w660] -> w640
                          tunnel: [w648 w659] -> w634
                          tunnel: [0.0 w658] -> w633
                          tunnel: [w648 w657] -> w630
                          tunnel: w628 -> [_ w654]
                          frame False {
                            w648 = dbl[] []
                          }
                          frame True {
                            n442 = Select(t=1.0, s=w654, f=0.0) -> (s? t:f=w653:dbl)
                            n443 = script code="optimization_main_loop"("syringe_pump"=w653) -> ("Conditions_Array"=w659:dbl[], "opt_ctr"=w660:dbl, "P_tot"=w658:dbl, "tau_array"=w657:dbl[], "experiment_history"=w655:dbl[][])  [unwired: 1 in, 1 out]
                            n444 = call-poly <vilib>:"Array To Matrix.vi"("Real 2D Array"=w655) -> ("Real Matrix"=w656:T18)
                            n445 = local write "experiment history"(w656) -> ()
                          }
                        }
                        "P_tot" <- w633
                        n446 = local read "COMM Port :: Milligat Pumps"() -> (w641:refnum<visa-resource-name>)
                        n447 = Equal?(x=w640, y=1.0) -> (x = y?=w638:bool)
                        n448 = flat-sequence {
                          tunnel: w634 -> [w1105]
                          tunnel: w630 -> [w1099]
                          frame #0 {
                            # "Start recording data"
                            n449 = Index Array(array=w1105, index=5) -> (element=w1117:dbl)
                            n450 = Index Array(array=w1105, index=0) -> (element=w1112:dbl)
                            n451 = Index Array(array=w1105, index=1) -> (element=w1113:dbl)
                            n452 = Index Array(array=w1105, index=2) -> (element=w1115:dbl)
                            n453 = Index Array(array=w1105, index=3) -> (element=w1114:dbl)
                            n454 = Index Array(array=w1105, index=4) -> (element=w1116:dbl)
                            n455 = local write "Pump setpoint(ul/min) 2"(w1113) -> ()
                            n456 = local write "Pump setpoint(ul/min) 4"(w1115) -> ()
                            n457 = local write "Pump setpoint(ul/min) 5"(w1116) -> ()
                            n458 = local write "Pump setpoint(ul/min) 3"(w1114) -> ()
                            n459 = local write "Pump setpoint(ul/min) 6"(w1117) -> ()
                            n460 = local write "Pump setpoint(ul/min) 1"(w1112) -> ()
                            n461 = Index Array(array=w1099, index=0) -> (element=w1104:dbl)
                            n462 = Index Array(array=w1099, index=4) -> (element=w1103:dbl)
                            n463 = Index Array(array=w1099, index=3) -> (element=w1102:dbl)
                            n464 = Index Array(array=w1099, index=2) -> (element=w1101:dbl)
                            n465 = Index Array(array=w1099, index=1) -> (element=w1100:dbl)
                            n466 = local write "tau 2"(w1100) -> ()
                            n467 = local write "tau 3"(w1101) -> ()
                            n468 = local write "tau 4"(w1102) -> ()
                            n469 = local write "tau 5"(w1103) -> ()
                            n470 = local write "tau 1"(w1104) -> ()
                          }
                        }
                        n471 = flat-sequence {
                          tunnel: w641 -> [w664]
                          tunnel: w634 -> [w663]
                          tunnel: w638 -> [w662]
                          tunnel: [w662] -> w647
                          tunnel: w635 -> [w661]
                          tunnel: w647 -> [w813]
                          tunnel: [w813] -> w646
                          tunnel: w646 -> [w833]
                          tunnel: [w831] -> w645
                          tunnel: w634 -> [w857]
                          tunnel: w645 -> [w856]
                          tunnel: w629 -> [w855]
                          tunnel: [w1035] -> w644
                          tunnel: w644 -> [w1048]
                          tunnel: [w1048] -> w643
                          tunnel: w643 -> [w1056]
                          tunnel: [w1056] -> w642
                          tunnel: [w1093] -> w637
                          tunnel: w642 -> [w1093]
                          frame #0 {
                            # "Setup pump flowrates and temperature setpoints"
                            n472 = stacked-sequence {
                              tunnel: w664 -> [w687 _ _ _ _]
                              tunnel: w664 -> [_ w728 _ _ _]
                              tunnel: w664 -> [_ _ w753 _ _]
                              tunnel: w664 -> [_ _ _ w778 _]
                              tunnel: w664 -> [_ _ _ _ w803]
                              tunnel: w663 -> [w684 w726 w751 w776 w800]
                              tunnel: w662 -> [w674 w719 w744 w769 w794]
                              tunnel: w661 -> [w672 _ _ _ _]
                              frame #0 {
                                # "Bay 1"
                                n473 = local read "Syringe_pump?"() -> (w673:bool)
                                n474 = Index Array(array=w684, index=0) -> (element=w682:dbl)
                                n475 = local read "BAY 1"() -> (w667:u16)
                                n476 = Index Array(array=w684, index=1) -> (element=w681:dbl)
                                n477 = Index Array(array=w684, index=6) -> (element=w680:dbl)
                                n478 = script code="MATLAB script"("T1_SP"=w680) -> ()  [unwired: 1 in, 1 out]
                                n479 = Less Or Equal?(x=w667, y=u16 4) -> (x <= y?=w669:bool)
                                n480 = Greater Or Equal?(x=w667, y=u16 1) -> (x >= y?=w670:bool)
                                n481 = And(x=w670, y=w669) -> (x .and. y?=w671:bool)
                                n482 = Greater Than 0?(x=w682) -> (x > 0?=w679:bool)
                                n483 = And(x=w679, y=w674) -> (x .and. y?=w678:bool)
                                n484 = Greater Than 0?(x=w681) -> (x > 0?=w677:bool)
                                n485 = Wait (ms)(milliseconds to wait=u32 300) -> ()  [unwired: 1 out]
                                n486 = And(x=w677, y=w674) -> (x .and. y?=w676:bool)
                                n487 = And(x=w671, y=w674) -> (x .and. y?=w675:bool)
                                n488 = case shown="False" w673 {
                                tunnel: w687 -> [w690 _]
                                tunnel: w681 -> [w689 w695]
                                tunnel: w676 -> [w688 w696]
                                tunnel: w672 -> [_ w694]
                                frame False {
                                n489 = case shown="False" w688 {
                                tunnel: w690 -> [w692 _]
                                tunnel: w689 -> [w691 _]
                                frame False {
                                n490 = call "PumpDispense.vi"("Flowrate(ul/min)"=w691, "Pump Address"="j", "Pump COMM Port"=w692) -> ()  [unwired: 7 in, 2 out]
                                }
                                frame True {
                                }
                                }
                                }
                                frame True {
                                n491 = case shown="False" w696 {
                                tunnel: w695 -> [_ w698]
                                tunnel: w694 -> [w697 w699]
                                frame False {
                                n492 = call <instrlib>:"Stop Pump.vi"("VISA resource name"=w697) -> ()  [unwired: 9 in, 2 out]
                                }
                                frame True {
                                w700 = u16 0 items=["Infuse", "Withdraw"] ("Run Direction (0:Infuse)")
                                w701 = u32 4 items=["milliliters per hour (ml/hr)", "milliliters per minute (ml/min)", "milliliters per second (ml/sec)", "microliters per hour (ul/hr)", "microliters per minute (ul/min)", "microliters per second (ul/sec)", "nanoliters per hour (nl/hr)", "nanoliters per minute (nl/min)", "nanoliters per second (nl/sec)", "picoliters per hour (pl/hr)", "picoliters per minute (pl/min)", "picoliters per second (pl/sec)"] ("Flow Rate Units (1:ml/min)")
                                w702 = u16 0 items=["Infuse", "Withdraw"] ("Pump Direction (0:Infuse)")
                                n493 = call <instrlib>:"Configure Flow Rate & Direction.vi"("VISA resource name"=w699, "Pump Direction (0:Infuse)"=w702, "Flow Rate (5.00)"=w698, "Flow Rate Units (1:ml/min)"=w701) -> ("VISA resource name out"=w703:refnum<visa-resource-name>)  [unwired: 10 in, 1 out]
                                n494 = call <instrlib>:"Start Pump.vi"("Run Direction (0:Infuse)"=w700, "VISA resource name"=w703) -> ()  [unwired: 8 in, 2 out]
                                }
                                }
                                }
                                }
                                n495 = case shown="True" w678 {
                                tunnel: w687 -> [w707 w709]
                                tunnel: w682 -> [_ w710]
                                frame False {
                                n496 = call "PumpStop.vi"("Pump Address"="g", "Pump COMM Port"=w707) -> ()  [unwired: 9 in, 1 out]
                                }
                                frame True {
                                n497 = call "PumpDispense.vi"("Flowrate(ul/min)"=w710, "Pump Address"="g", "Pump COMM Port"=w709) -> ()  [unwired: 7 in, 2 out]
                                }
                                }
                                n498 = case shown="True" w675 {
                                tunnel: w680 -> [_ w706]
                                frame False {
                                n499 = local write "Temperature Control 1"(FALSE) -> ()
                                }
                                frame True {
                                n500 = local write "Temperature SP 1"(w706) -> ()
                                n501 = local write "Temperature Control 1"(TRUE ("Temperature Control 1")) -> ()
                                }
                                }
                              }
                              frame #1 {
                                # "Bay 2"
                                n502 = local read "BAY 2"() -> (w715:u16)
                                n503 = Index Array(array=w726, index=2) -> (element=w723:dbl)
                                n504 = Index Array(array=w726, index=7) -> (element=w724:dbl)
                                n505 = script code="MATLAB script"("T2_SP"=w724) -> ()  [unwired: 1 in, 1 out]
                                n506 = Greater Than 0?(x=w723) -> (x > 0?=w721:bool)
                                n507 = And(x=w721, y=w719) -> (x .and. y?=w720:bool)
                                n508 = Greater Or Equal?(x=w715, y=u16 1) -> (x >= y?=w713:bool)
                                n509 = Less Or Equal?(x=w715, y=u16 4) -> (x <= y?=w718:bool)
                                n510 = And(x=w713, y=w718) -> (x .and. y?=w717:bool)
                                n511 = And(x=w717, y=w719) -> (x .and. y?=w722:bool)
                                n512 = case shown="True" w722 {
                                tunnel: w724 -> [_ w735]
                                frame False {
                                n513 = local write "Temperature Control 2"(FALSE) -> ()
                                }
                                frame True {
                                n514 = local write "Temperature Control 2"(TRUE ("Temperature Control 2")) -> ()
                                n515 = local write "Temperature SP 2"(w735) -> ()
                                }
                                }
                                n516 = case shown="False" w720 {
                                tunnel: w723 -> [_ w731]
                                tunnel: w728 -> [w729 w732]
                                frame False {
                                n517 = call "PumpStop.vi"("Pump Address"="i", "Pump COMM Port"=w729) -> ()  [unwired: 9 in, 1 out]
                                }
                                frame True {
                                n518 = call "PumpDispense.vi"("Flowrate(ul/min)"=w731, "Pump Address"="i", "Pump COMM Port"=w732) -> ()  [unwired: 7 in, 2 out]
                                }
                                }
                                n519 = Wait (ms)(milliseconds to wait=u32 300) -> ()  [unwired: 1 out]
                              }
                              frame #2 {
                                # "Bay 3"
                                n520 = local read "BAY 3"() -> (w739:u16)
                                n521 = Index Array(array=w751, index=3) -> (element=w748:dbl)
                                n522 = Not Equal To 0?(x=w748) -> (x != 0?=w747:bool)
                                n523 = Index Array(array=w751, index=8) -> (element=w749:dbl)
                                n524 = script code="MATLAB script"("T3_SP"=w749) -> ()  [unwired: 1 in, 1 out]
                                n525 = Less Or Equal?(x=w739, y=u16 4) -> (x <= y?=w743:bool)
                                n526 = Greater Or Equal?(x=w739, y=u16 1) -> (x >= y?=w740:bool)
                                n527 = And(x=w740, y=w743) -> (x .and. y?=w738:bool)
                                n528 = And(x=w738, y=w744) -> (x .and. y?=w745:bool)
                                n529 = And(x=w747, y=w744) -> (x .and. y?=w746:bool)
                                n530 = case shown="True" w746 {
                                tunnel: w748 -> [_ w756]
                                tunnel: w753 -> [w754 w757]
                                frame False {
                                n531 = call "PumpStop.vi"("Pump Address"="e", "Pump COMM Port"=w754) -> ()  [unwired: 9 in, 1 out]
                                }
                                frame True {
                                n532 = call "PumpDispense.vi"("Flowrate(ul/min)"=w756, "Pump Address"="e", "Pump COMM Port"=w757) -> ()  [unwired: 7 in, 2 out]
                                }
                                }
                                n533 = case shown="False" w745 {
                                tunnel: w749 -> [_ w760]
                                frame False {
                                n534 = local write "Temperature Control 3"(FALSE) -> ()
                                }
                                frame True {
                                n535 = local write "Temperature Control 3"(TRUE ("Temperature Control 3")) -> ()
                                n536 = local write "Temperature SP 3"(w760) -> ()
                                }
                                }
                                n537 = Wait (ms)(milliseconds to wait=u32 300) -> ()  [unwired: 1 out]
                              }
                              frame #3 {
                                # "Bay 4"
                                n538 = Index Array(array=w776, index=9) -> (element=w773:dbl)
                                n539 = script code="MATLAB script"("T4_SP"=w773) -> ()  [unwired: 1 in, 1 out]
                                n540 = Index Array(array=w776, index=4) -> (element=w774:dbl)
                                n541 = Not Equal To 0?(x=w774) -> (x != 0?=w772:bool)
                                n542 = local read "BAY 4"() -> (w763:u16)
                                n543 = And(x=w772, y=w769) -> (x .and. y?=w771:bool)
                                n544 = Less Or Equal?(x=w763, y=u16 4) -> (x <= y?=w768:bool)
                                n545 = Greater Or Equal?(x=w763, y=u16 1) -> (x >= y?=w765:bool)
                                n546 = And(x=w765, y=w768) -> (x .and. y?=w764:bool)
                                n547 = And(x=w764, y=w769) -> (x .and. y?=w770:bool)
                                n548 = case shown="True" w771 {
                                tunnel: w778 -> [w779 w782]
                                tunnel: w774 -> [_ w781]
                                frame False {
                                n549 = call "PumpStop.vi"("Pump Address"="f", "Pump COMM Port"=w779) -> ()  [unwired: 9 in, 1 out]
                                }
                                frame True {
                                n550 = call "PumpDispense.vi"("Flowrate(ul/min)"=w781, "Pump Address"="f", "Pump COMM Port"=w782) -> ()  [unwired: 7 in, 2 out]
                                }
                                }
                                n551 = case shown="True" w770 {
                                tunnel: w773 -> [_ w785]
                                frame False {
                                n552 = local write "Temperature Control 4"(FALSE ("Temperature Control 4")) -> ()
                                }
                                frame True {
                                n553 = local write "Temperature SP 4"(w785) -> ()
                                n554 = local write "Temperature Control 4"(TRUE ("Temperature Control 5")) -> ()
                                }
                                }
                                n555 = Wait (ms)(milliseconds to wait=u32 300) -> ()  [unwired: 1 out]
                              }
                              frame #4 {
                                # "Bay 5"
                                n556 = Index Array(array=w800, index=5) -> (element=w798:dbl)
                                n557 = Index Array(array=w800, index=4) -> (element=w799:dbl)
                                n558 = script code="MATLAB script"("T5_SP"=w799) -> ()  [unwired: 1 in, 1 out]
                                n559 = local read "BAY 5"() -> (w789:u16)
                                n560 = Not Equal To 0?(x=w798) -> (x != 0?=w796:bool)
                                n561 = And(x=w796, y=w794) -> (x .and. y?=w795:bool)
                                n562 = Less Or Equal?(x=w789, y=u16 4) -> (x <= y?=w793:bool)
                                n563 = Greater Or Equal?(x=w789, y=u16 1) -> (x >= y?=w790:bool)
                                n564 = case shown="False" w795 {
                                tunnel: w803 -> [w804 w807]
                                tunnel: w798 -> [_ w806]
                                frame False {
                                n565 = call "PumpStop.vi"("Pump Address"="h", "Pump COMM Port"=w804) -> ()  [unwired: 9 in, 1 out]
                                }
                                frame True {
                                n566 = call "PumpDispense.vi"("Flowrate(ul/min)"=w806, "Pump Address"="h", "Pump COMM Port"=w807) -> ()  [unwired: 7 in, 2 out]
                                }
                                }
                                n567 = And(x=w790, y=w793) -> (x .and. y?=w788:bool)
                                n568 = And(x=w788, y=w794) -> (x .and. y?=w797:bool)
                                n569 = case shown="True" w797 {
                                tunnel: w799 -> [_ w810]
                                frame False {
                                n570 = local write "Temperature Control 5"(FALSE ("Temperature Control 5")) -> ()
                                }
                                frame True {
                                n571 = local write "Temperature SP 5"(w810) -> ()
                                n572 = local write "Temperature Control 5"(TRUE ("Temperature Control 5")) -> ()
                                }
                                }
                                n573 = Wait (ms)(milliseconds to wait=u32 300) -> ()  [unwired: 1 out]
                              }
                            }
                          }
                          frame #1 {
                            # "Wait till Steady State temperature readings on all bays"
                            n574 = while {
                              tunnel: w813 -> [w814]
                              stop <- w815 stop-if-true
                              n575 = flat-sequence {
                                tunnel: [w818] -> w815
                                tunnel: w814 -> [w817]
                                frame #0 {
                                n576 = Wait (ms)(milliseconds to wait=u32 1500) -> ()  [unwired: 1 out]
                                }
                                frame #1 {
                                n577 = local read "Temp SS? 2"() -> (w821:bool)
                                n578 = local read "Temp SS? 3"() -> (w822:bool)
                                n579 = local read "Temp SS? 4"() -> (w823:bool)
                                n580 = local read "Temp SS? 5"() -> (w824:bool)
                                n581 = local read "Temp SS? 1"() -> (w820:bool)
                                n582 = Not(x=w817) -> (.not. x?=w830:bool)
                                n583 = local read "Stop"() -> (w819:bool)
                                n584 = And(x=w822, y=w823) -> (x .and. y?=w826:bool)
                                n585 = And(x=w820, y=w821) -> (x .and. y?=w827:bool)
                                n586 = And(x=w827, y=w826) -> (x .and. y?=w825:bool)
                                n587 = And(x=w825, y=w824) -> (x .and. y?=w828:bool)
                                n588 = Or(x=w830, y=w828) -> (x .or. y?=w829:bool)
                                n589 = Or(x=w829, y=w819) -> (x .or. y?=w818:bool)
                                }
                              }
                            }
                            n590 = local write "Calculate condition"(TRUE ("Calculate condition")) -> ()
                          }
                          frame #2 {
                            n591 = flat-sequence {
                              tunnel: w833 -> [w835]
                              tunnel: [w835] -> w832
                              tunnel: w832 -> [w842]
                              tunnel: [w842] -> w831
                              frame #0 {
                                n592 = local write "Equlibrating Temperature"(TRUE) -> ()
                              }
                              frame #1 {
                                # "Wait 1.5 system volumes"
                                n593 = local read "Number of System Flushes per condtion"() -> (w839:dbl)
                                n594 = local read "Extra system dead volume"() -> (w840:dbl)
                                n595 = script code="start = tic;\nP_tot = P1+P2+P3+P4+P5+P6;\nif P_tot >0\n  extra_res = extr_sys_dead_vol/P_tot;\nelse\n   extra_res =0;\nend\ntotal_sys_res = tau1 + tau2 + tau3 + tau4 + tau5 + extra_res;\ntotal_wait_time = total_sys_res*num_flush_per_cond*60;"("extr_sys_dead_vol"=w840, "num_flush_per_cond"=w839) -> ("??"=w843:errorcluster, "total_wait_time"=w837:dbl, "total_sys_res"=→"Total System Resisdence Time(min)":dbl)  [unwired: 1 in]
                                n596 = Divide(x=w837, y=60.0) -> (x/y=→"total_flush_time":dbl)
                                n597 = while {
                                tunnel: w842 -> [w845]
                                tunnel: w843 -> [w848]
                                stop <- w849 stop-if-true
                                # "Check if system is flushed every 10 seconds"
                                n598 = script code="end1 = toc(start);\nflush_time = 0;\nif end1 > total_wait_time\n   flush_time = 1;\nend\ncurr_wait_time = end1 /60;"("??"=w848) -> ("flush_time"=w852:dbl, "curr_wait_time"=w847:dbl)  [unwired: 1 out]
                                "curr_wait_time" <- w847
                                n599 = Not Equal To 0?(x=w852) -> (x != 0?=w851:bool)
                                n600 = Multiply(x=60.0, y=w847) -> ()  [unwired: 1 out]
                                n601 = local read "Stop"() -> (w854:bool)
                                n602 = Or(x=w851, y=w854) -> (x .or. y?=w850:bool)
                                n603 = Not(x=w845) -> (.not. x?=w844:bool)
                                n604 = Wait (ms)(milliseconds to wait=u32 10000) -> ()  [unwired: 1 out]
                                n605 = Or(x=w850, y=w844) -> (x .or. y?=w849:bool)
                                }
                              }
                            }
                          }
                          frame #3 {
                            # "Collect HPLC Data"
                            n606 = flat-sequence {
                              tunnel: w857 -> [w866]
                              tunnel: w856 -> [w865]
                              tunnel: w855 -> [w864]
                              tunnel: w855 -> [w863]
                              frame #0 {
                                n607 = local read "pause for ms"() -> (w860:bool)
                                n608 = case shown="True" w860 {
                                frame False {
                                }
                                frame True {
                                n609 = One Button Dialog(message="Press OK to Analyze Data", button name ("OK")="OK" ("Left Button Text (\"Yes\")")) -> ()  [unwired: 1 out]
                                }
                                }
                                n610 = local write "Flushing System"(TRUE ("Flushing System")) -> ()
                                "System Flushed?" <- TRUE ("System Flushed?")
                              }
                              frame #1 {
                                n611 = flat-sequence {
                                tunnel: w866 -> [w871]
                                tunnel: w865 -> [_]
                                tunnel: w864 -> [w870]
                                tunnel: w863 -> [w869]
                                frame #0 {
                                }
                                frame #1 {
                                n612 = flat-sequence {
                                tunnel: w871 -> [w873]
                                tunnel: w870 -> [w950]
                                tunnel: w871 -> [_]
                                tunnel: [w970] -> w868
                                tunnel: [w969] -> w867
                                tunnel: w869 -> [w968]
                                tunnel: w868 -> [w1003]
                                tunnel: w867 -> [w1002]
                                frame #0 {
                                n613 = local read "COMM Port :: Milligat Pumps"() -> (w875:refnum<visa-resource-name>)
                                n614 = stacked-sequence {
                                tunnel: w875 -> [w883 w895 w913 w918 w927 w940]
                                tunnel: w873 -> [w882 w891 w910 w920 w929 w936]
                                tunnel: 1.0 ("Flowrate(ul/min)") -> [w881 w890 w908 w917 w926 w935]
                                frame #0 {
                                n615 = Index Array(array=w882, index=0) -> (element=w885:dbl)
                                n616 = Greater Than 0?(x=w885) -> (x > 0?=w884:bool)
                                n617 = case shown="True" w884 {
                                tunnel: w883 -> [_ w888]
                                tunnel: w881 -> [_ w887]
                                frame False {
                                }
                                frame True {
                                n618 = call "PumpDispense.vi"("Flowrate(ul/min)"=w887, "Pump Address"="g", "Pump COMM Port"=w888) -> ()  [unwired: 7 in, 2 out]
                                }
                                }
                                }
                                frame #1 {
                                n619 = Index Array(array=w891, index=1) -> (element=w893:dbl)
                                n620 = Greater Than 0?(x=w893) -> (x > 0?=w892:bool)
                                n621 = case shown="False" w892 {
                                tunnel: w890 -> [_ w897]
                                tunnel: w895 -> [_ w896]
                                frame False {
                                }
                                frame True {
                                n622 = local read "Syringe_pump?"() -> (w898:bool)
                                n623 = case shown="False" w898 {
                                tunnel: w897 -> [w899 _]
                                tunnel: w896 -> [w900 _]
                                frame False {
                                n624 = call "PumpDispense.vi"("Flowrate(ul/min)"=w899, "Pump Address"="j", "Pump COMM Port"=w900) -> ()  [unwired: 7 in, 2 out]
                                }
                                frame True {
                                w907 = u16 0 items=["Infuse", "Withdraw"] ("Run Direction (0:Infuse)")
                                w903 = u32 4 items=["milliliters per hour (ml/hr)", "milliliters per minute (ml/min)", "milliliters per second (ml/sec)", "microliters per hour (ul/hr)", "microliters per minute (ul/min)", "microliters per second (ul/sec)", "nanoliters per hour (nl/hr)", "nanoliters per minute (nl/min)", "nanoliters per second (nl/sec)", "picoliters per hour (pl/hr)", "picoliters per minute (pl/min)", "picoliters per second (pl/sec)"] ("Flow Rate Units (1:ml/min)")
                                w904 = u16 0 items=["Infuse", "Withdraw"] ("Pump Direction (0:Infuse)")
                                n625 = local read "COMM Port:: Harvard Syringe Pump"() -> (w905:refnum<visa-resource-name>)
                                n626 = call <instrlib>:"Configure Flow Rate & Direction.vi"("VISA resource name"=w905, "Pump Direction (0:Infuse)"=w904, "Flow Rate (5.00)"=i8 2 ("Pump Address"), "Flow Rate Units (1:ml/min)"=w903) -> ("VISA resource name out"=w906:refnum<visa-resource-name>)  [unwired: 10 in, 1 out]
                                n627 = call <instrlib>:"Start Pump.vi"("Run Direction (0:Infuse)"=w907, "VISA resource name"=w906) -> ()  [unwired: 8 in, 2 out]
                                }
                                }
                                }
                                }
                                }
                                frame #2 {
                                n628 = Index Array(array=w910, index=2) -> (element=w911:dbl)
                                n629 = Greater Than 0?(x=w911) -> (x > 0?=w909:bool)
                                n630 = case shown="True" w909 {
                                tunnel: w913 -> [_ w915]
                                tunnel: w908 -> [_ w914]
                                frame False {
                                }
                                frame True {
                                n631 = call "PumpDispense.vi"("Flowrate(ul/min)"=w914, "Pump Address"="i", "Pump COMM Port"=w915) -> ()  [unwired: 7 in, 2 out]
                                }
                                }
                                }
                                frame #3 {
                                n632 = Index Array(array=w920, index=3) -> (element=w921:dbl)
                                n633 = Greater Than 0?(x=w921) -> (x > 0?=w919:bool)
                                n634 = case shown="True" w919 {
                                tunnel: w918 -> [_ w924]
                                tunnel: w917 -> [_ w923]
                                frame False {
                                }
                                frame True {
                                n635 = call "PumpDispense.vi"("Flowrate(ul/min)"=w923, "Pump Address"="e", "Pump COMM Port"=w924) -> ()  [unwired: 7 in, 2 out]
                                }
                                }
                                }
                                frame #4 {
                                n636 = Index Array(array=w929, index=4) -> (element=w930:dbl)
                                n637 = Greater Than 0?(x=w930) -> (x > 0?=w928:bool)
                                n638 = case shown="True" w928 {
                                tunnel: w927 -> [_ w933]
                                tunnel: w926 -> [_ w932]
                                frame False {
                                }
                                frame True {
                                n639 = call "PumpDispense.vi"("Flowrate(ul/min)"=w932, "Pump Address"="f", "Pump COMM Port"=w933) -> ()  [unwired: 7 in, 2 out]
                                }
                                }
                                }
                                frame #5 {
                                n640 = Index Array(array=w936, index=5) -> (element=w938:dbl)
                                n641 = Greater Than 0?(x=w938) -> (x > 0?=w937:bool)
                                n642 = case shown="True" w937 {
                                tunnel: w940 -> [_ w942]
                                tunnel: w935 -> [_ w941]
                                frame False {
                                }
                                frame True {
                                n643 = call "PumpDispense.vi"("Flowrate(ul/min)"=w941, "Pump Address"="h", "Pump COMM Port"=w942) -> ()  [unwired: 7 in, 2 out]
                                }
                                }
                                }
                                }
                                n644 = stacked-sequence {
                                tunnel: FALSE -> [w876 w877 w878 w879 w880]
                                frame #0 {
                                n645 = local write "Temperature Control 1"(w876) -> ()
                                }
                                frame #1 {
                                n646 = local write "Temperature Control 2"(w877) -> ()
                                }
                                frame #2 {
                                n647 = local write "Temperature Control 3"(w878) -> ()
                                }
                                frame #3 {
                                n648 = local write "Temperature Control 4"(w879) -> ()
                                }
                                frame #4 {
                                n649 = local write "Temperature Control 5"(w880) -> ()
                                }
                                }
                                }
                                frame #1 {
                                n650 = while {
                                stop <- w949 stop-if-true
                                n651 = local read "Phase_Sensor_voltage"() -> (w944:dbl)
                                n652 = script code="organic_phase = 0;\nif start_phase_time \n   start_phase_timer = tic;\n   start_phase_time = 0;\nelse\n  %ignore phase sensor values\n  %if not(phase_sensor_val >2.9 && phase_sensor_val <3.8)\n    %    start_phase_timer = tic;\n   %end\n\n   end_phase_time =  toc(start_phase_timer )\n\n   if end_phase_time > 2\n       organic_phase = 1;\n       start_phase_time = 1;\n   end\n\nend"("phase_sensor_val"=w944) -> ("organic_phase"=w946:dbl)  [unwired: 1 in, 1 out]
                                n653 = local read "Stop"() -> (w948:bool)
                                n654 = Not Equal To 0?(x=w946) -> (x != 0?=w947:bool)
                                n655 = Or(x=w947, y=w948) -> (x .or. y?=w949:bool)
                                n656 = Wait (ms)(milliseconds to wait=u32 300) -> ()  [unwired: 1 out]
                                }
                                }
                                frame #2 {
                                n657 = local read "Stop"() -> (w952:bool)
                                n658 = Not(x=w952) -> (.not. x?=w951:bool)
                                n659 = local read "Sample Valve COMM::Port"() -> (w953:refnum<visa-resource-name>)
                                n660 = case shown="True" w951 {
                                tunnel: w953 -> [_ w955]
                                tunnel: w950 -> [_ w954]
                                frame False {
                                }
                                frame True {
                                n661 = flat-sequence {
                                tunnel: w954 -> [w957]
                                tunnel: w955 -> [w967]
                                frame #0 {
                                n662 = local read "Sample Valve COMM::Port"() -> (w956:refnum<visa-resource-name>)
                                n663 = flat-sequence {
                                tunnel: w959 -> [w964]
                                tunnel: [w964] -> w958
                                frame #0 {
                                n664 = Wait (ms)(milliseconds to wait=u32 500) -> ()  [unwired: 1 out]
                                }
                                }
                                n665 = call-poly <vilib>:"Digital Write.vi"("Output Value"=FALSE, "DO Channel"=u8 22, "LINX Resource"=w958) -> ()  [unwired: 7 in, 2 out]
                                n666 = call-poly <vilib>:"Digital Write.vi"("Output Value"=TRUE, "DO Channel"=u8 22, "LINX Resource"=w957) -> ("LINX Resource"=w959:T10)  [unwired: 7 in, 1 out]
                                n667 = call "NanoValve Inject.vi"("VISA resource name"=w956) -> ()  [unwired: 10 in, 1 out]
                                }
                                frame #1 {
                                n668 = Wait (ms)(milliseconds to wait=u32 2000) -> ()  [unwired: 1 out]
                                }
                                frame #2 {
                                n669 = call "NanoValve Load.vi"("VISA resource name"=w967) -> ()  [unwired: 10 in, 1 out]
                                }
                                }
                                }
                                }
                                }
                                frame #3 {
                                n670 = local read "Stop"() -> (w973:bool)
                                n671 = local read "Bay Parameters"() -> (w969:T2)
                                n672 = Unbundle By Name(w969) -> ("Hplc Wait time(min)"=w971:dbl)
                                n673 = Not(x=w973) -> (.not. x?=w972:bool)
                                n674 = case shown="True" w972 {
                                tunnel: w971 -> [_ w978]
                                tunnel: [errorcluster {"status"=FALSE, "code"=0, "source"=""} ("error out") w977] -> w970
                                tunnel: w969 -> [_ w976]
                                tunnel: w968 -> [_ w975]
                                frame False {
                                }
                                frame True {
                                n675 = flat-sequence {
                                tunnel: w978 -> [w980]
                                tunnel: w975 -> [w989]
                                tunnel: [w1000] -> w977
                                tunnel: w976 -> [w999]
                                frame #0 {
                                # "Wait till for HPLC Method"
                                n676 = script code="start = tic;"() -> ("??"=w979:errorcluster)  [unwired: 1 in]
                                n677 = while {
                                tunnel: w980 -> [w982]
                                tunnel: w979 -> [w981]
                                stop <- w988 stop-if-true
                                n678 = Multiply(x=w982, y=60.0) -> (x*y=w983:dbl)
                                n679 = script code="end1 = toc(start);\nflush_time = 0;\nif end1 > hplc_wait_time\n   flush_time = 1;\nend"("??"=w981, "hplc_wait_time"=w983) -> ("flush_time"=w985:dbl)  [unwired: 1 out]
                                n680 = local read "Stop"() -> (w987:bool)
                                n681 = Not Equal To 0?(x=w985) -> (x != 0?=w986:bool)
                                n682 = Or(x=w986, y=w987) -> (x .or. y?=w988:bool)
                                }
                                }
                                frame #1 {
                                n683 = flat-sequence {
                                tunnel: w991 -> [w996]
                                tunnel: [w996] -> w990
                                frame #0 {
                                n684 = Wait (ms)(milliseconds to wait=u32 500) -> ()  [unwired: 1 out]
                                }
                                }
                                n685 = call-poly <vilib>:"Digital Write.vi"("Output Value"=FALSE, "DO Channel"=u8 24, "LINX Resource"=w989) -> ("LINX Resource"=w991:T10)  [unwired: 7 in, 1 out]
                                n686 = call-poly <vilib>:"Digital Write.vi"("Output Value"=TRUE, "DO Channel"=u8 24, "LINX Resource"=w990) -> ()  [unwired: 7 in, 2 out]
                                }
                                frame #2 {
                                n687 = Wait (ms)(milliseconds to wait=u32 30000) -> ()  [unwired: 1 out]
                                }
                                frame #3 {
                                n688 = Unbundle By Name(w999) -> ("hplc File Name"=w1001:string)
                                n689 = call "hplc_analyze.vi"("File Path"=w1001) -> ("error out"=w1000:errorcluster)  [unwired: 10 in]
                                }
                                }
                                }
                                }
                                }
                                frame #4 {
                                n690 = Unbundle By Name(w1003) -> ("status"=w1004:bool)
                                n691 = case shown="False" w1004 {
                                tunnel: w1002 -> [_ w1005]
                                frame False {
                                }
                                frame True {
                                n692 = while {
                                tunnel: w1005 -> [w1007]
                                stop <- w1006 stop-if-true
                                w1012 = "An error occured while trying to read HPLC data. " ("message")
                                n693 = local write "Error Message"(w1012) -> ()
                                n694 = call <vilib>:"Three Button Dialog.vi"("Right Button Text (\"Cancel\")"="STOP EXPs" ("F button name (\"Cancel\")"), "Center Button Text (\"No\")"="REDO" ("T button name (\"OK\")"), "Left Button Text (\"Yes\")"="REREAD" ("T button name (\"OK\")"), "message"=w1012) -> ("Which Button?"=w1008:T19)  [unwired: 7 in]
                                n695 = case shown="\"Left Button\"" w1008 {
                                tunnel: w1007 -> [_ _ w1019 _]
                                tunnel: [TRUE TRUE w1018 w1021] -> w1006
                                frame "Right Button" {
                                w1013 = TRUE ("Setup Error")
                                n696 = local write "System Error"(w1013) -> ()
                                n697 = local write "Setup Error"(w1013) -> ()
                                n698 = script code="system_error = 1"() -> ()  [unwired: 1 in, 1 out]
                                n699 = local write "Stop"(w1013) -> ()
                                }
                                frame "Center Button" {
                                n700 = script code="redo = true;\nopt_ctr = 1;\nCurrExp = CurrExp + 1;\nncall0 = ncall0 +1;\nif req_ctr == req_tot\n       opt_ctr = 3;\n  else\n     req_ctr = req_ctr +1;\nend"() -> ()  [unwired: 1 in, 1 out]
                                }
                                frame "Left Button" {
                                n701 = Unbundle By Name(w1019) -> ("hplc File Name"=w1020:string)
                                n702 = call "hplc_analyze.vi"("File Path"=w1020) -> ("error out"=w1016:errorcluster)  [unwired: 10 in]
                                n703 = Unbundle By Name(w1016) -> ("status"=w1017:bool)
                                n704 = Not(x=w1017) -> (.not. x?=w1018:bool)
                                }
                                frame "Window Close" {
                                w1021 = TRUE
                                n705 = local write "Setup Error"(w1021) -> ()
                                n706 = script code="system_error = 1"() -> ()  [unwired: 1 in, 1 out]
                                n707 = local write "Stop"(w1021) -> ()
                                }
                                }
                                }
                                }
                                }
                                }
                                frame #5 {
                                n708 = disable-structure shown="Disabled" {
                                frame Disabled {
                                n709 = flat-sequence {
                                tunnel: w1023 -> [w1028]
                                tunnel: [w1028] -> w1022
                                frame #0 {
                                n710 = Wait (ms)(milliseconds to wait=u32 500) -> ()  [unwired: 1 out]
                                }
                                }
                                n711 = call-poly <vilib>:"Digital Write.vi"("Output Value"=FALSE, "DO Channel"=u8 22) -> ("LINX Resource"=w1023:T10)  [unwired: 8 in, 1 out]
                                n712 = call-poly <vilib>:"Digital Write.vi"("Output Value"=TRUE, "DO Channel"=u8 22, "LINX Resource"=w1022) -> ()  [unwired: 7 in, 2 out]
                                }
                                frame Enabled {
                                }
                                }
                                }
                                }
                                }
                                }
                              }
                              frame #2 {
                                n713 = local read "Stop"() -> (w1031:bool)
                                n714 = local write "HPLC Analysis"(TRUE ("HPLC Analysis")) -> ()
                                n715 = Not(x=w1031) -> (.not. x?=w1030:bool)
                                n716 = case shown="True" w1030 {
                                frame False {
                                }
                                frame True {
                                n717 = script code="C_measured =Conc;\nFvalues(end +1,:) = [Conc];"() -> ()  [unwired: 1 in, 1 out]
                                }
                                }
                              }
                            }
                          }
                          frame #4 {
                            n718 = local read "Stop"() -> (w1034:bool)
                            n719 = Not(x=w1034) -> (.not. x?=w1033:bool)
                            n720 = case shown="True" w1033 {
                              tunnel: [1.0 w1045] -> w1035
                              frame False {
                              }
                              frame True {
                                # "Save data to excel file"
                                n721 = local read "Bay Parameters"() -> (w1043:T2)
                                n722 = Unbundle By Name(w1043) -> ("Total Number of Experiments 2"=w1042:dbl)
                                n723 = script code="analyze_labview_results"("ncall"=w1042) -> ("terminate"=w1045:dbl, "ncall0"=w1044:dbl, "experiment_history"=w1040:dbl[][], "Pbest"=w1038:dbl[], "Tbest"=w1039:dbl[], "best_exp_num"=w1037:dbl)  [unwired: 1 in, 1 out]
                                n724 = local write "Flowrates(ul/min)_best"(w1038) -> ()
                                n725 = local write "temperature_best"(w1039) -> ()
                                n726 = local write "best_exp_num"(w1037) -> ()
                                n727 = local write "Current Experiment"(w1044) -> ()
                                n728 = local write "Total Number of Experiments"(w1042) -> ()
                                n729 = call-poly <vilib>:"Array To Matrix.vi"("Real 2D Array"=w1040) -> ("Real Matrix"=w1041:T18)
                                n730 = local write "experiment history"(w1041) -> ()
                              }
                            }
                          }
                          frame #5 {
                            n731 = local read "Num_exp_till_pause"() -> (w1047:i32)
                            n732 = Increment(x=w1047) -> (x+1=w1046:i32)
                            n733 = local write "Num_exp_till_pause"(w1046) -> ()
                          }
                          frame #6 {
                            # "Pause System"
                            n734 = local read "Bay Parameters"() -> (w1055:T2)
                            n735 = Unbundle By Name(w1055) -> ("Num_conditons_per_wait"=w1054:dbl)
                            n736 = local read "Num_exp_till_pause"() -> (w1053:i32)
                            n737 = Equal?(x=w1054, y=w1053) -> (x = y?=w1052:bool)
                            n738 = local read "Run_Stop_cluster"() -> (w1049:T7)
                            n739 = Unbundle By Name(w1049) -> ("Stop Run Button"=w1051:bool)
                            n740 = Or(x=w1051, y=w1052) -> (x .or. y?=w1050:bool)
                            n741 = case shown="True" w1050 {
                              tunnel: w1054 -> [w1058 _]
                              tunnel: w1053 -> [w1059 _]
                              tunnel: w1049 -> [_ w1061]
                              frame False {
                                n742 = Greater?(x=w1059, y=w1058) -> (0:w1057:bool)
                                n743 = case shown="True" w1057 {
                                frame False {
                                }
                                frame True {
                                n744 = local write "Num_exp_till_pause"(0 ("Num_exp_till_pause")) -> ()
                                }
                                }
                              }
                              frame True {
                                n745 = flat-sequence {
                                tunnel: w1061 -> [w1089]
                                frame #0 {
                                w1065 = string[] ["e", "f", "g", "h", "i", "j"]
                                # "Turn off pumps and stop controling temperature"
                                n746 = stacked-sequence {
                                frame #0 {
                                n747 = local write "Temperature Control 1"(FALSE ("Temperature Control 1")) -> ()
                                }
                                frame #1 {
                                n748 = local write "Temperature Control 2"(FALSE ("Temperature Control 2")) -> ()
                                }
                                frame #2 {
                                n749 = local write "Temperature Control 3"(FALSE ("Temperature Control 3")) -> ()
                                }
                                frame #3 {
                                n750 = local write "Temperature Control 4"(FALSE ("Temperature Control 4")) -> ()
                                }
                                frame #4 {
                                n751 = local write "Temperature Control 5"(FALSE ("Temperature Control 5")) -> ()
                                }
                                }
                                n752 = local read "COMM Port:: Harvard Syringe Pump"() -> (w1063:refnum<visa-resource-name>)
                                n753 = local read "Syringe_pump?"() -> (w1062:bool)
                                n754 = local read "COMM Port :: Milligat Pumps"() -> (w1064:refnum<visa-resource-name>)
                                n755 = Array Size(array=w1065) -> (size(s)=w1066:i32)
                                n756 = case shown="True" w1062 {
                                tunnel: w1063 -> [_ w1074]
                                frame False {
                                }
                                frame True {
                                n757 = call <instrlib>:"Stop Pump.vi"("VISA resource name"=w1074) -> ()  [unwired: 9 in, 2 out]
                                }
                                }
                                n758 = for {
                                N: w1066 -> [_]
                                tunnel: w1065 -> [w1072] mode=indexing
                                tunnel: w1064 -> [w1073]
                                n759 = call "PumpStop.vi"("Pump Address"=w1072, "Pump COMM Port"=w1073) -> ()  [unwired: 9 in, 1 out]
                                }
                                }
                                frame #1 {
                                n760 = local read "Stop"() -> (w1077:bool)
                                n761 = Not(x=w1077) -> (.not. x?=w1076:bool)
                                n762 = case shown="True" w1076 {
                                frame False {
                                }
                                frame True {
                                n763 = while {
                                stop <- w1083 stop-if-true
                                # "Wait till user confirms system resume"
                                n764 = Two Button Dialog(message="System is currently paused. Refill Syringes, flush lines, then press OK to continue optimization.\nOr Redo to repeat condition ", 1:"REDO" ("F button name (\"Cancel\")"), 2:"OK" ("Left Button Text (\"Yes\")")) -> (T button?=w1079:bool)
                                n765 = case shown="False" w1079 {
                                tunnel: [TRUE TRUE] -> w1078
                                frame False {
                                n766 = script code="redo = true;"() -> ()  [unwired: 1 in, 1 out]
                                }
                                frame True {
                                }
                                }
                                n767 = local read "Stop"() -> (w1084:bool)
                                n768 = Or(x=w1078, y=w1084) -> (x .or. y?=w1083:bool)
                                }
                                }
                                }
                                n769 = local write "stop_xl_write"(TRUE ("stop_xl_write")) -> ()
                                }
                                frame #2 {
                                n770 = local write "Num_exp_till_pause"(0 ("Num_exp_till_pause")) -> ()
                                n771 = Bundle By Name(cluster=w1089, "Stop Run Button"=FALSE) -> (w1087:T7)
                                n772 = local write "Run_Stop_cluster"(w1087) -> ()
                                }
                                }
                              }
                            }
                          }
                          frame #7 {
                            w1092 = FALSE
                            n773 = local write "Equlibrating Temperature"(w1092) -> ()
                            n774 = local write "Calculate condition"(w1092) -> ()
                            n775 = local write "Flushing System"(w1092) -> ()
                            n776 = local write "HPLC Analysis"(w1092) -> ()
                            n777 = local write "stop_xl_write"(TRUE ("stop_xl_write")) -> ()
                          }
                        }
                        n778 = while {
                          stop <- w1119 stop-if-true
                          n779 = flat-sequence {
                            frame #0 {
                              n780 = script code="save_excel_time_data;"() -> ()  [unwired: 1 in, 1 out]
                            }
                            frame #1 {
                              n781 = Wait (ms)(milliseconds to wait=u32 30000) -> ()  [unwired: 1 out]
                            }
                          }
                          n782 = local read "Stop"() -> (w1120:bool)
                          n783 = local read "stop_xl_write"() -> (w1118:bool)
                          n784 = Or(x=w1118, y=w1120) -> (x .or. y?=w1119:bool)
                        }
                      }
                    }
                  }
                }
                n785 = Greater?(x=w602, y=w603) -> (0:w610:bool)
                n786 = Equal?(x=w608, y=1.0) -> (x = y?=w604:bool)
                n787 = local read "Stop"() -> (w611:bool)
                n788 = Or(x=w611, y=w610) -> (x .or. y?=w607:bool)
                n789 = Or(x=w604, y=w607) -> (x .or. y?=w606:bool)
                n790 = case shown="True" w604 {
                  frame False {
                  }
                  frame True {
                    w615 = u16 2 items=["System  Error", "System Running", "System Standby"] ("System Status")
                    n791 = local write "Stop"(TRUE ("Stop")) -> ()
                    n792 = local write "System Status"(w615) -> ()
                  }
                }
                "Optimization_loop_index" <- w612
              }
            }
          }
          n793 = while {
            tunnel: w590 -> [w1215]
            stop <- w1218 stop-if-true
            n794 = local read "Temperature Control 3"() -> (w1216:bool)
            n795 = local read "running?"() -> (w1214:bool)
            n796 = And(x=w1214, y=w1216) -> (x .and. y?=w1217:bool)
            n797 = case shown="True" w1217 {
              tunnel: w1215 -> [_ w1221]
              frame False {
                n798 = local write "Temp SS? 3"(TRUE) -> ()
              }
              frame True {
                # "Bay 3 Temperature Controller"
                n799 = local read "Temperature SP 3"() -> (w1222:dbl)
                n800 = local read "Temperature 3"() -> (w1225:dbl)
                n801 = Subtract(x=w1225, y=w1222) -> (x-y=w1234:dbl)
                n802 = Absolute Value(x=w1234) -> (abs(x)=w1236:dbl)
                n803 = Less Or Equal?(x=w1236, y=1.2) -> (x <= y?=w1233:bool)
                n804 = local write "Temp SS? 3"(w1233) -> ()
                n805 = local read "SSR Duration 3"() -> (w1243:dbl)
                n806 = call-poly <vilib>:"PID Online Autotuning.vi"("setpoint"=w1222, "manipulated variable"=w1243, "autotuning parameters"=T9 {"type of controller"=enum."PID", "relay cycles"=3, "relay amplitude"=1.0, "control specifications"=enum."Normal", "PV noise level"=0.1} ("Autotuning Parameters R1"), "process variable"=w1225, "PID gains in"=T8 {"Proportional gain Kc"=0.38538, "Integral time Ti (sec)"=0.524375, "Derivative time Ti (sec)"=0.12585} ("PID gains 2")) -> ("setpoint out"=w1241:dbl, "process variable out"=w1242:dbl, "PID gains out"=w1245:T17)  [unwired: 6 in, 2 out]
                n807 = Greater?(x=w1222, y=w1225) -> (0:w1232:bool)
                n808 = call <vilib>:"PID Autotuning (Temperature).vi"("desired temperature"=w1241, "measured temperature"=w1242, "PID gains in"=w1245, "output range"=cluster{"output high":dbl, "output low":dbl} {"output high"=3.0, "output low"=-1.0} ("Output range")) -> ("output"=w1238:dbl)  [unwired: 12 in, 3 out]
                n809 = Multiply(x=1000.0, y=w1238) -> (x*y=w1240:dbl)
                n810 = local write "SSR Duration 3"(w1238) -> ()
                n811 = Greater Than 0?(x=w1240) -> (x > 0?=w1231:bool)
                n812 = And(x=w1231, y=w1232) -> (x .and. y?=w1229:bool)
                n813 = Subtract(x=w1225, y=10.0) -> (x-y=w1227:dbl)
                n814 = Less?(x=w1227, y=w1222) -> (x < y?=w1230:bool)
                n815 = And(x=w1230, y=w1229) -> (x .and. y?=w1228:bool)
                n816 = case shown="True" w1228 {
                  tunnel: [errorcluster {"status"=FALSE, "code"=0, "source"=""} ("error out") w1257] -> _
                  tunnel: 4 -> [_ w1255]
                  tunnel: w1240 -> [w1251 w1256]
                  tunnel: [0.0 w1259] -> w1223
                  tunnel: w1222 -> [_ w1258]
                  tunnel: w1221 -> [_ w1254]
                  frame False {
                    n817 = Absolute Value(x=w1251) -> (abs(x)=w1252:dbl)
                    n818 = Wait (ms)(milliseconds to wait=w1252) -> ()  [unwired: 1 out]
                  }
                  frame True {
                    n819 = call "TurnOnRelayArduino.vi"("channel"=w1255, "duration"=w1256, "LINX Resource"=w1254) -> ("error out"=w1257:errorcluster)  [unwired: 7 in, 1 out]
                    n820 = script code="tempdiff3= SP3 - T3;\nif tempdiff3 > 10\n  if slope3 < .01\n     temp_check3 = temp_check3 + 1;\n  else\n      temp_check3 =0;\n  end\nend\n\nif temp_check3 > 9\n  temp_error3 = 1\nend"("SP3"=w1258) -> ("temp_error3"=w1259:dbl)  [unwired: 1 in, 1 out]
                  }
                }
                n821 = Not Equal To 0?(x=w1223) -> (x != 0?=w1224:bool)
                n822 = case shown="True" w1224 {
                  frame False {
                  }
                  frame True {
                    n823 = local write "Error Message"("Bay 3 Temperature Heating Error") -> ()
                  }
                }
                n824 = case shown="True" w1224 {
                  tunnel: w1224 -> [_ w1249]
                  frame False {
                  }
                  frame True {
                    n825 = local write "System Error"(w1249) -> ()
                    n826 = local write "Stop"(w1249) -> ()
                  }
                }
              }
            }
            n827 = Wait (ms)(milliseconds to wait=u32 400) -> ()  [unwired: 1 out]
            n828 = local read "Stop"() -> (w1218:bool)
          }
          n829 = while {
            tunnel: w590 -> [w1169]
            stop <- w1172 stop-if-true
            n830 = local read "running?"() -> (w1168:bool)
            n831 = Wait (ms)(milliseconds to wait=u32 400) -> ()  [unwired: 1 out]
            n832 = local read "Temperature Control 4"() -> (w1171:bool)
            n833 = And(x=w1168, y=w1171) -> (x .and. y?=w1170:bool)
            n834 = case shown="True" w1170 {
              tunnel: w1169 -> [_ w1175]
              frame False {
                n835 = local write "Temp SS? 4"(TRUE ("Temp SS? 4")) -> ()
              }
              frame True {
                # "Bay 4 Temperature Controller"
                n836 = local read "Temperature SP 4"() -> (w1178:dbl)
                n837 = local read "Temperature 4"() -> (w1181:dbl)
                n838 = Subtract(x=w1181, y=w1178) -> (x-y=w1188:dbl)
                n839 = Absolute Value(x=w1188) -> (abs(x)=w1190:dbl)
                n840 = Less Or Equal?(x=w1190, y=1.2) -> (x <= y?=w1187:bool)
                n841 = local write "Temp SS? 4"(w1187) -> ()
                n842 = local read "SSR Duration 4"() -> (w1191:dbl)
                n843 = call-poly <vilib>:"PID Online Autotuning.vi"("setpoint"=w1178, "manipulated variable"=w1191, "autotuning parameters"=T9 {"type of controller"=enum."PID", "relay cycles"=3, "relay amplitude"=1.0, "control specifications"=enum."Normal", "PV noise level"=0.1} ("Autotuning Parameters R1"), "process variable"=w1181, "PID gains in"=T8 {"Proportional gain Kc"=0.38538, "Integral time Ti (sec)"=0.524375, "Derivative time Ti (sec)"=0.12585} ("PID gains 2")) -> ("setpoint out"=w1193:dbl, "process variable out"=w1194:dbl, "PID gains out"=w1196:T17)  [unwired: 6 in, 2 out]
                n844 = call <vilib>:"PID Autotuning (Temperature).vi"("desired temperature"=w1193, "measured temperature"=w1194, "PID gains in"=w1196, "output range"=cluster{"output high":dbl, "output low":dbl} {"output high"=3.0, "output low"=-1.0} ("Output range")) -> ("output"=w1192:dbl)  [unwired: 12 in, 3 out]
                n845 = Subtract(x=w1181, y=10.0) -> (x-y=w1180:dbl)
                n846 = Less?(x=w1180, y=w1178) -> (x < y?=w1182:bool)
                n847 = Multiply(x=1000.0, y=w1192) -> (x*y=w1200:dbl)
                n848 = Greater?(x=w1178, y=w1181) -> (0:w1186:bool)
                n849 = Greater Than 0?(x=w1200) -> (x > 0?=w1185:bool)
                n850 = local write "SSR Duration 4"(w1192) -> ()
                n851 = And(x=w1185, y=w1186) -> (x .and. y?=w1184:bool)
                n852 = And(x=w1182, y=w1184) -> (x .and. y?=w1183:bool)
                n853 = case shown="True" w1183 {
                  tunnel: [errorcluster {"status"=FALSE, "code"=0, "source"=""} ("error out") w1211] -> _
                  tunnel: 5 -> [_ w1209]
                  tunnel: w1200 -> [w1205 w1210]
                  tunnel: w1178 -> [_ w1213]
                  tunnel: [0.0 w1212] -> w1177
                  tunnel: w1175 -> [_ w1208]
                  frame False {
                    n854 = Absolute Value(x=w1205) -> (abs(x)=w1206:dbl)
                    n855 = Wait (ms)(milliseconds to wait=w1206) -> ()  [unwired: 1 out]
                  }
                  frame True {
                    n856 = call "TurnOnRelayArduino.vi"("channel"=w1209, "duration"=w1210, "LINX Resource"=w1208) -> ("error out"=w1211:errorcluster)  [unwired: 7 in, 1 out]
                    n857 = script code="tempdiff4= SP4 - T4;\nif tempdiff4 > 10\n  if slope4 < .01\n     temp_check4 = temp_check4 + 1;\n  else\n      temp_check4 =0;\n  end\nend\n\nif temp_check4 > 9\n  temp_error4 = 1\nend"("SP4"=w1213) -> ("temp_error4"=w1212:dbl)  [unwired: 1 in, 1 out]
                  }
                }
                n858 = Not Equal To 0?(x=w1177) -> (x != 0?=w1176:bool)
                n859 = case shown="True" w1176 {
                  frame False {
                  }
                  frame True {
                    n860 = local write "Error Message"("Bay 4 Temperature Heating Error") -> ()
                  }
                }
                n861 = case shown="True" w1176 {
                  tunnel: w1176 -> [_ w1203]
                  frame False {
                  }
                  frame True {
                    n862 = local write "System Error"(w1203) -> ()
                    n863 = local write "Stop"(w1203) -> ()
                  }
                }
              }
            }
            n864 = local read "Stop"() -> (w1172:bool)
          }
          n865 = while {
            stop <- w595 stop-if-true
            n866 = script code="TempArr1=circshift(TempArr1,9);\nTempArr2=circshift(TempArr2,9);\nTempArr3=circshift(TempArr3,9);\nTempArr4=circshift(TempArr4,9);\nTempArr5=circshift(TempArr5,9);\n\nTempArr1(10)=T1;\nTempArr2(10)=T2;\nTempArr3(10)=T3;\nTempArr4(10)=T4;\nTempArr5(10)=T5;\n\n[slope1 temp] = polyfit([1,2,3,4,5,6,7,8,9,10]',TempArr1,1);\nslope1 = slope1(1);\n[slope2 temp] = polyfit([1,2,3,4,5,6,7,8,9,10]',TempArr2,1);\nslope2= slope2(1);\n[slope3 temp] = polyfit([1,2,3,4,5,6,7,8,9,10]',TempArr3,1);\nslope3 = slope3(1);\n[slope4 temp] = polyfit([1,2,3,4,5,6,7,8,9,10]',TempArr4,1);\nslope4 = slope4(1);\n[slope5 temp] = polyfit([1,2,3,4,5,6,7,8,9,10]',TempArr5,1);\nslope5 = slope5(1);"() -> ()  [unwired: 1 in, 1 out]
            n867 = Wait (ms)(milliseconds to wait=u32 600) -> ()  [unwired: 1 out]
            n868 = local read "Stop"() -> (w595:bool)
          }
          n869 = while {
            tunnel: w590 -> [w1123]
            stop <- w1126 stop-if-true
            n870 = local read "running?"() -> (w1122:bool)
            n871 = local read "Temperature Control 5"() -> (w1124:bool)
            n872 = And(x=w1122, y=w1124) -> (x .and. y?=w1125:bool)
            n873 = case shown="True" w1125 {
              tunnel: w1123 -> [_ w1129]
              frame False {
                n874 = local write "Temp SS? 5"(TRUE ("Temp SS? 5")) -> ()
              }
              frame True {
                # "Bay 5 Temperature Controller"
                n875 = local read "SSR Duration 5"() -> (w1145:dbl)
                n876 = local read "Temperature SP 5"() -> (w1131:dbl)
                n877 = local read "Temperature 5"() -> (w1134:dbl)
                n878 = Subtract(x=w1134, y=w1131) -> (x-y=w1142:dbl)
                n879 = Absolute Value(x=w1142) -> (abs(x)=w1144:dbl)
                n880 = Less Or Equal?(x=w1144, y=1.2) -> (x <= y?=w1141:bool)
                n881 = local write "Temp SS? 5"(w1141) -> ()
                n882 = call-poly <vilib>:"PID Online Autotuning.vi"("setpoint"=w1131, "manipulated variable"=w1145, "autotuning parameters"=T9 {"type of controller"=enum."PID", "relay cycles"=3, "relay amplitude"=1.0, "control specifications"=enum."Normal", "PV noise level"=0.1} ("Autotuning Parameters R1"), "process variable"=w1134, "PID gains in"=T8 {"Proportional gain Kc"=0.38538, "Integral time Ti (sec)"=0.524375, "Derivative time Ti (sec)"=0.12585} ("PID gains 2")) -> ("setpoint out"=w1147:dbl, "process variable out"=w1148:dbl, "PID gains out"=w1150:T17)  [unwired: 6 in, 2 out]
                n883 = call <vilib>:"PID Autotuning (Temperature).vi"("desired temperature"=w1147, "measured temperature"=w1148, "PID gains in"=w1150, "output range"=cluster{"output high":dbl, "output low":dbl} {"output high"=3.0, "output low"=-1.0} ("Output range")) -> ("output"=w1146:dbl)  [unwired: 12 in, 3 out]
                n884 = Multiply(x=1000.0, y=w1146) -> (x*y=w1154:dbl)
                n885 = Greater?(x=w1131, y=w1134) -> (0:w1139:bool)
                n886 = Greater Than 0?(x=w1154) -> (x > 0?=w1140:bool)
                n887 = local write "SSR Duration 5"(w1146) -> ()
                n888 = And(x=w1140, y=w1139) -> (x .and. y?=w1137:bool)
                n889 = Subtract(x=w1134, y=10.0) -> (x-y=w1135:dbl)
                n890 = Greater?(x=w1135, y=w1131) -> (0:w1138:bool)
                n891 = And(x=w1138, y=w1137) -> (x .and. y?=w1136:bool)
                n892 = case shown="True" w1136 {
                  tunnel: [errorcluster {"status"=FALSE, "code"=0, "source"=""} ("error out") w1165] -> _
                  tunnel: 6 -> [_ w1162]
                  tunnel: w1154 -> [w1159 w1163]
                  tunnel: [0.0 w1167] -> w1132
                  tunnel: w1131 -> [_ w1166]
                  tunnel: w1129 -> [_ w1164]
                  frame False {
                    n893 = Absolute Value(x=w1159) -> (abs(x)=w1160:dbl)
                    n894 = Wait (ms)(milliseconds to wait=w1160) -> ()  [unwired: 1 out]
                  }
                  frame True {
                    n895 = call "TurnOnRelayArduino.vi"("channel"=w1162, "duration"=w1163, "LINX Resource"=w1164) -> ("error out"=w1165:errorcluster)  [unwired: 7 in, 1 out]
                    n896 = script code="tempdiff5= SP5 - T5;\n\nif tempdiff5 > 10\n  if slope5 < .01\n     temp_check5 = temp_check5 + 1;\n  else\n      temp_check5 =0;\n  end\nend\n\nif temp_check5 >9\n  temp_error5 = 1\nend"("SP5"=w1166) -> ("temp_error5"=w1167:dbl)  [unwired: 1 in, 1 out]
                  }
                }
                n897 = Not Equal To 0?(x=w1132) -> (x != 0?=w1130:bool)
                n898 = case shown="True" w1130 {
                  frame False {
                  }
                  frame True {
                    n899 = local write "Error Message"("Bay 5 Temperature Heating Error") -> ()
                  }
                }
                n900 = case shown="True" w1130 {
                  tunnel: w1130 -> [_ w1157]
                  frame False {
                  }
                  frame True {
                    n901 = local write "Stop"(w1157) -> ()
                    n902 = local write "System Error"(w1157) -> ()
                  }
                }
              }
            }
            n903 = Wait (ms)(milliseconds to wait=u32 400) -> ()  [unwired: 1 out]
            n904 = local read "Stop"() -> (w1126:bool)
          }
        }
      }
      n905 = local read "IR Sensor Device"() -> (w62:T6)
      n906 = while {
        tunnel: errorcluster {"status"=FALSE, "code"=0, "source"=""} ("error out") -> [w133]
        tunnel: w62 -> [w152]
        stop <- w173 stop-if-true
        w130 = u8 7 items=["RAM IR raw  Ch1"=4, "RAM IR raw  Ch2"=5, "RAM T_A"=6, "RAM T_OBJ1"=7, "RAM T_OBJ2"=8, "EEPROM_To_max"=32, "EEPROM_To_min"=33, "EEPROM_PWM_CTRL"=34, "EEPROM_Ta_range"=35, "EEPROM_Emissivity_CorrCoeff"=36, "EEPROM_SMBus Address"=46, "EEPROM_ConfigReg"=37] ("Melexis_Cmmds")
        # "Bay 5 Temperature Read"
        # "Bay 4 Temperature Read"
        # "Bay 3 Temperature Read"
        # "Bay 2 Temperature Read"
        # "Bay 1 Temperature Read"
        n907 = local read "Stop"() -> (w173:bool)
        n908 = call "IRSensorNIRead.vi"("error in (no error)"=w133, "Melexis_Cmmds"=w130, "Address"=u8 1, "device reference"=w152) -> ("error out"=w155:errorcluster, "Temperature"=w153:dbl, "device reference out"=w151:T6)  [unwired: 5 in]
        n909 = local write "error out"(w155) -> ()
        n910 = Unbundle By Name(w155) -> ("status"=w154:bool)
        n911 = call-poly <vilib>:"PID Control Input Filter.vi"("input"=w153) -> ("output"=w166:dbl)  [unwired: 4 in]
        n912 = case shown="False" w154 {
          tunnel: w165 -> [w182 _]
          tunnel: [w182 w183] -> w170
          frame False {
            n913 = local write "Temperature 1"(w182) -> ()
          }
          frame True {
            n914 = local read "Temperature 1"() -> (w183:dbl)
          }
        }
        n915 = flat-sequence {
          tunnel: w166 -> [w196]
          tunnel: [w196] -> w165
          tunnel: w151 -> [w195]
          tunnel: [w195] -> w150
          frame #0 {
            n916 = Wait (ms)(milliseconds to wait=u32 100) -> ()  [unwired: 1 out]
          }
        }
        n917 = call "IRSensorNIRead.vi"("error in (no error)"=w133, "Melexis_Cmmds"=w130, "Address"=u8 2, "device reference"=w150) -> ("error out"=w142:errorcluster, "Temperature"=w143:dbl, "device reference out"=w145:T6)  [unwired: 5 in]
        n918 = local write "error out"(w142) -> ()
        n919 = Unbundle By Name(w142) -> ("status"=w147:bool)
        n920 = call-poly <vilib>:"PID Control Input Filter.vi"("input"=w143) -> ("output"=w164:dbl)  [unwired: 4 in]
        n921 = case shown="True" w147 {
          tunnel: w163 -> [w180 _]
          tunnel: [w180 w181] -> w169
          frame False {
            n922 = local write "Temperature 2"(w180) -> ()
          }
          frame True {
            n923 = local read "Temperature 2"() -> (w181:dbl)
          }
        }
        n924 = flat-sequence {
          tunnel: w164 -> [w193]
          tunnel: [w193] -> w163
          tunnel: w145 -> [w192]
          tunnel: [w192] -> w144
          frame #0 {
            n925 = Wait (ms)(milliseconds to wait=u32 100) -> ()  [unwired: 1 out]
          }
        }
        n926 = call "IRSensorNIRead.vi"("error in (no error)"=w133, "Melexis_Cmmds"=w130, "Address"=u8 3, "device reference"=w144) -> ("error out"=w135:errorcluster, "Temperature"=w141:dbl, "device reference out"=w140:T6)  [unwired: 5 in]
        n927 = local write "error out"(w135) -> ()
        n928 = Unbundle By Name(w135) -> ("status"=w136:bool)
        n929 = case shown="False" w136 {
          tunnel: w160 -> [w178 _]
          tunnel: [w178 w179] -> w162
          frame False {
            n930 = local write "Temperature 3"(w178) -> ()
          }
          frame True {
            n931 = local read "Temperature 3"() -> (w179:dbl)
          }
        }
        n932 = call-poly <vilib>:"PID Control Input Filter.vi"("input"=w141) -> ("output"=w161:dbl)  [unwired: 4 in]
        n933 = flat-sequence {
          tunnel: w161 -> [w190]
          tunnel: [w190] -> w160
          tunnel: w140 -> [w189]
          tunnel: [w189] -> w138
          frame #0 {
            n934 = Wait (ms)(milliseconds to wait=u32 100) -> ()  [unwired: 1 out]
          }
        }
        n935 = call "IRSensorNIRead.vi"("error in (no error)"=w133, "Melexis_Cmmds"=w130, "Address"=u8 4, "device reference"=w138) -> ("error out"=w125:errorcluster, "Temperature"=w137:dbl, "device reference out"=w132:T6)  [unwired: 5 in]
        n936 = local write "error out"(w125) -> ()
        n937 = Unbundle By Name(w125) -> ("status"=w127:bool)
        n938 = case shown="True" w127 {
          tunnel: w158 -> [w176 _]
          tunnel: [w176 w177] -> w168
          frame False {
            n939 = local write "Temperature 4"(w176) -> ()
          }
          frame True {
            n940 = local read "Temperature 4"() -> (w177:dbl)
          }
        }
        n941 = call-poly <vilib>:"PID Control Input Filter.vi"("input"=w137) -> ("output"=w159:dbl)  [unwired: 4 in]
        n942 = flat-sequence {
          tunnel: w159 -> [w187]
          tunnel: [w187] -> w158
          tunnel: w132 -> [w186]
          tunnel: [w186] -> w131
          frame #0 {
            n943 = Wait (ms)(milliseconds to wait=u32 100) -> ()  [unwired: 1 out]
          }
        }
        n944 = call "IRSensorNIRead.vi"("error in (no error)"=w133, "Melexis_Cmmds"=w130, "Address"=u8 5, "device reference"=w131) -> ("error out"=w128:errorcluster, "Temperature"=w129:dbl)  [unwired: 5 in, 1 out]
        n945 = local write "error out"(w128) -> ()
        n946 = flat-sequence {
          tunnel: w157 -> [w184]
          tunnel: [w184] -> w156
          frame #0 {
            n947 = Wait (ms)(milliseconds to wait=u32 100) -> ()  [unwired: 1 out]
          }
        }
        n948 = Unbundle By Name(w128) -> ("status"=w126:bool)
        n949 = call-poly <vilib>:"PID Control Input Filter.vi"("input"=w129) -> ("output"=w157:dbl)  [unwired: 4 in]
        n950 = local write "error out"(w133) -> ()
        n951 = Build Array(w170, w169, w162, w168, w156) -> (w172:dbl[])
        n952 = Array To Cluster(array=w172) -> (cluster=→"Teperature Chart":T3)
        n953 = case shown="False" w126 {
          tunnel: w156 -> [w174 _]
          tunnel: [w174 w175] -> w167
          frame False {
            n954 = local write "Temperature 5"(w174) -> ()
          }
          frame True {
            n955 = local read "Temperature 5"() -> (w175:dbl)
          }
        }
        n956 = script code="MATLAB script"("T1"=w170, "T2"=w169, "T3"=w162, "T4"=w168, "T5"=w167) -> ()  [unwired: 1 in, 1 out]
      }
      n957 = while {
        stop <- w88 stop-if-true
        n958 = local read "Pump setpoint(ul/min) 1"() -> (w91:dbl)
        n959 = local read "Pump setpoint(ul/min) 2"() -> (w87:dbl)
        n960 = local read "Pump setpoint(ul/min) 3"() -> (w86:dbl)
        n961 = local read "Pump setpoint(ul/min) 4"() -> (w85:dbl)
        n962 = local read "Pump setpoint(ul/min) 5"() -> (w84:dbl)
        n963 = local read "Pump setpoint(ul/min) 6"() -> (w83:dbl)
        n964 = Build Array(w91, w87, w86, w85, w84, w83) -> (w92:dbl[])
        n965 = Array To Cluster(array=w92) -> (cluster=→"Pump Setpoints Chart":T3)
        n966 = Wait (ms)(milliseconds to wait=u32 5000) -> ()  [unwired: 1 out]
        n967 = local read "Stop"() -> (w88:bool)
      }
      n968 = while {
        stop <- w70 stop-if-true
        n969 = local read "System Error"() -> (w69:bool)
        n970 = Wait (ms)(milliseconds to wait=u32 300) -> ()  [unwired: 1 out]
        n971 = case shown="True" w69 {
          tunnel: [w74 w75] -> w67
          frame False {
            w71 = u16 2 items=["System  Error", "System Running", "System Standby"] ("System Status")
            w72 = u16 1 items=["System  Error", "System Running", "System Standby"] ("System Status")
            n972 = local read "running?"() -> (w73:bool)
            n973 = Select(t=w72, s=w73, f=w71) -> (s? t:f=w74:u16)
          }
          frame True {
            w75 = u16 0 items=["System  Error", "System Running", "System Standby"] ("System Status")
          }
        }
        n974 = local read "Stop"() -> (w70:bool)
        n975 = local write "System Status"(w67) -> ()
      }
      n976 = while {
        tunnel: w61 -> [w76]
        stop <- w82 stop-if-true
        n977 = call-poly <vilib>:"Analog Read.vi"("Analog Channel"=u8 0, "LINX Resource"=w76) -> ("Voltage"=w77:dbl)  [unwired: 6 in, 3 out]
        "Phase_Sensor_voltage" <- w77
        n978 = Wait (ms)(milliseconds to wait=u32 300) -> ()  [unwired: 1 out]
        n979 = Build Array(w77) -> (w79:dbl[])
        n980 = Array To Cluster(array=w79) -> (cluster=→"Phase Sensor Chart":T3)
        n981 = local read "Stop"() -> (w82:bool)
      }
      n982 = while {
        tunnel: w61 -> [w95]
        stop <- w120 stop-if-true
        w102 = 270
        w96 = 600
        w97 = 600
        # "Read Pressure and Flowrate"
        n983 = local read "Stop"() -> (w120:bool)
        n984 = call-poly <vilib>:"Analog Read.vi"("AI Channel(s)"=i32[] [14, 15, 14, 15], "LINX Resource"=w95) -> ("Voltages"=w93:dbl[])  [unwired: 6 in, 3 out]
        n985 = Index Array(array=w93, index=1) -> (element=w116:dbl)
        n986 = Index Array(array=w93, index=0) -> (element=w117:dbl)
        n987 = call-poly <vilib>:"PID Control Input Filter.vi"("input"=w116) -> ("output"=w109:dbl)  [unwired: 4 in]
        n988 = call-poly <vilib>:"PID Control Input Filter.vi"("input"=w117) -> ("output"=w108:dbl)  [unwired: 4 in]
        n989 = Multiply(x=104.96 ("y"), y=w109) -> (x*y=w110:dbl)
        n990 = Multiply(x=104.96 ("y"), y=w108) -> (x*y=w113:dbl)
        n991 = Subtract(x=w110, y=24.077) -> (x-y=w100:dbl)
        n992 = Subtract(x=w113, y=24.077) -> (x-y=w101:dbl)
        n993 = Build Array(w97, w96) -> (w105:i32[])
        n994 = Array To Cluster(array=w105) -> (cluster=→"Flowrate Chart":T4)
        n995 = Build Array(w101, w100) -> (w106:dbl[])
        n996 = local write "Flowrate Sensor 1"(w97) -> ()
        n997 = local write "Flowrate Sensor 2"(w96) -> ()
        n998 = local write "Pressure 1"(w101) -> ()
        n999 = local write "Pressure 2"(w100) -> ()
        n1000 = Array To Cluster(array=w106) -> (cluster=→"Pressure Chart":T3)
        n1001 = Wait (ms)(milliseconds to wait=u32 500) -> ()  [unwired: 1 out]
        n1002 = script code="MATLAB script"("F1"=w97, "F2"=w96, "Pres1"=w101, "Pres2"=w100) -> ()  [unwired: 1 in, 1 out]
        n1003 = Greater?(x=w100, y=w102) -> (0:w98:bool)
        n1004 = Greater?(x=w101, y=w102) -> (0:w99:bool)
        n1005 = case shown="True" w99 {
          frame False {
          }
          frame True {
            w124 = TRUE ("Stop")
            n1006 = local write "System Error"(w124) -> ()
            n1007 = local write "Stop"(w124) -> ()
            n1008 = local write "Error Message"("Pressure Sensor 1 readings above 250psi") -> ()
            n1009 = script code="system_error = 1;"() -> ()  [unwired: 1 in, 1 out]
          }
        }
        n1010 = case shown="False" w98 {
          frame False {
          }
          frame True {
            w122 = TRUE ("Stop")
            n1011 = local write "System Error"(w122) -> ()
            n1012 = local write "Error Message"("Pressure Sensor 2 readings above 250psi") -> ()
            n1013 = local write "Stop"(w122) -> ()
            n1014 = script code="system_error = 1;"() -> ()  [unwired: 1 in, 1 out]
          }
        }
      }
    }
    frame #3 {
      # "Save and close xml and excel file"
      n1015 = script code="if exist('xl_file','var') & exist('xlApp','var')\n  xlWorkbook.SaveAs(xl_file);\n  xlWorkbook.Close;\n  xlApp.Quit;\n  xlApp.delete;\nend"() -> ()  [unwired: 1 in, 1 out]
    }
    frame #4 {
      w1363 = string[] ["e", "f", "g", "h", "i", "j"]
      # "End communication to hardware"
      n1016 = local read "Syringe_pump?"() -> (w1361:bool)
      n1017 = local read "COMM Port:: Harvard Syringe Pump"() -> (w1362:refnum<visa-resource-name>)
      n1018 = local read "IR Sensor Device"() -> (w1360:T6)
      n1019 = local read "COMM Port :: Milligat Pumps"() -> (w1365:refnum<visa-resource-name>)
      n1020 = call <vilib>:"Close.vi"("LINX Resource"=w1359) -> ()  [unwired: 10 in, 1 out]
      n1021 = Array Size(array=w1363) -> (size(s)=w1364:i32)
      n1022 = case shown="True" w1361 {
        tunnel: w1362 -> [_ w1366]
        frame False {
        }
        frame True {
          n1023 = call <instrlib>:"Stop Pump.vi"("VISA resource name"=w1366) -> ()  [unwired: 9 in, 2 out]
        }
      }
      n1024 = for {
        N: w1364 -> [_]
        tunnel: w1363 -> [w1367] mode=indexing
        tunnel: w1365 -> [w1368]
        n1025 = call "PumpStop.vi"("Pump Address"=w1367, "Pump COMM Port"=w1368) -> ()  [unwired: 9 in, 1 out]
        n1026 = Wait (ms)(milliseconds to wait=u32 300) -> ()  [unwired: 1 out]
      }
      n1027 = call-poly <vilib>:"NI-845x Close Reference.vi"("device reference"=w1360) -> ()  [unwired: 10 in, 1 out]
    }
    frame #5 {
      # "Display Error Messages if necessary"
      n1028 = local read "Error Message"() -> (w1370:string)
      n1029 = One Button Dialog(message=w1370) -> ()  [unwired: 1 in, 1 out]
    }
  }
